vi "Dashboard Main.vi"() -> ()   [LabVIEW 2014]
uses:
  Common Code/Elevator DB Control.ctl
  Common Code/Elevator Presets.ctl
  Common Code/Roller Indicators.ctl
  Common Code/Roller Mode Enum.ctl
  Common Code/Auto Roller Commands.ctl
  Common Code/Inner Roller States.ctl
  Robot Code/Sensors/Pot Data.ctl
  Robot Code/Rollers/Untip Can States.ctl
  Common Code/Roller Control.ctl
  <vilib>/Rock Robotics/WPI/Camera/WPI_CameraSettings Read MJPG.ctl
  <vilib>/Rock Robotics/WPI/Camera/WPI_CameraImageSize.ctl
  Common Code/Encoder Control.ctl
  Common Code/Encoder Values SuperCluster.ctl
  Common Code/Encoder Values.ctl
  Common Code/Power and Diagnostic Data.ctl
  Common Code/Utilities/PDP Data.ctl
  Common Code/Utilities/PCM Data.ctl
  Common Code/Loop Timings.ctl
  Common Code/Ultrasonic Indicators.ctl
  Common Code/Drivetrain Status.ctl
  Robot Code/Drivetrain Code/Drivetrain Mode.ctl
  Common Code/Dist Drive Status.ctl
  Common Code/Yaw Rate Compensation Indicators.ctl
  <vilib>/vision/Image Controls.llb/IMAQ Image.ctl
  Vision/Particle Filter Settings.ctl
  Robot Code/Rollers/ThinRollerIndicators.ctl
  Vision/Vision Tote Data.ctl
  Common Code/commandCluster.ctl
  Common Code/Drivetrain Settings.ctl
  Common Code/IMU Data.ctl
  navX-MXP Library/COMMON/TypeDefs/Value TypeDefs/navX NAVX_CAL_STATUS.ctl
  navX-MXP Library/COMMON/TypeDefs/Value TypeDefs/navX NAVX_OP_STATUS.ctl
  Common Code/Elevator Status.ctl
  Common Code/Elevator Mode.ctl
  Common Code/Auto Elevator Indicators.ctl
  Common Code/Elevator State.ctl
  Robot Code/Pike/Pike Indicators.ctl
  Robot Code/Pike/Pike State.ctl
  Robot Code/Pike/Pike Mode.ctl
  <vilib>/Utility/miscctls.llb/LVPointTypeDef.ctl
  Common Code/Dashboard Control Data.ctl
  Robot Code/Pike/Pike DB Controls.ctl
  Common Code/Dashboard Display Data.ctl
  Common Code/AutonomousDBPacket.ctl
  <vilib>/Rock Robotics/WPI/Dashboard/WPI_DashboardLogging Global.vi
  <vilib>/picture/picture.llb/Draw True-Color Pixmap.vi
  <vilib>/Utility/config.llb/Write Key (String).vi
  <vilib>/Utility/config.llb/Write Key (I32).vi
  <vilib>/Utility/inputDevices.llb/keyboardAcquire.vi
  <vilib>/Utility/config.llb/NI_LVConfig.lvlib
  navX-MXP Library/navX-MXP IMU.lvlib
panel:
  out "Axis Cam":T1
  out "DumbDash Message":string
  in  "Load":bool
  in  "Save":bool
  in  "stop":bool
  in  "TCP":refnum<k5>
  in  "Rec Mode":enum32{"Stop", "Record", "Playback"}(radio)
  out "Camera IP":string
  out "Image Message":string="Timeout in Camera Communications"
  in  "Dashboard Tab":T2(tab)
  out "Pike":bool
  in  "Dallas load":bool
  out "Stabilizer":bool
  out "Finger":bool
  out "NAVX_CAL_STATUS":T3 items=["IMU_CAL_STATE_MASK"=3, "IMU_CAL_INPROGRESS"=0, "IMU_CAL_ACCUMULATE"=1, "IMU_CAL_COMPLETE"=2, "MAG_CAL_COMPLETE"=4, "BARO_CAL_COMPLETE"=8]
  out "Elevator View 2":picture
  out "Trashcan? 2":bool caption="Trashcan?"
  out "Robot Mode":T4(ring)=enum."Auto Disabled"
  out "Gyro":dbl(knob) scale=0.0..360.0 scale format="%#.7g"
  out "Roller Indicators":T5={"Rollers Closed?"=FALSE, "Zero Complete?"=FALSE, "Roller Mode"=enum."Manual", "Auto Roller State"=enum."Grab Tote", "Intake State"=enum."Acquire Tote", "Left Out"=0.0, "Roller Safety Open"=FALSE, "Right Out"=0.0} {"Right Out" scale=-1.0..1.0; "Left Out" scale=-1.0..1.0}
  out "Elevator Mode":bool
  out "Roller Mode":bool
  out "Pressure":dbl format="%#.1f"
  out "Ultrasonic Data 2":T9
  out "Auton File":string
  out "Elevator Status Data 2":T10 {"Finger Raw" format="%#.3f"; "Finger Height" format="%#.3f"; "Motor Out" scale=-1.0..1.0}
  out "Robot IP":string
  out "Pike Indicators":T14={"Motor Out"=0.0, "Current"=0.0, "Limit Switch"=FALSE, "Current Limit"=FALSE, "State"=enum."Going Up", "Command"=enum."Auto Up"}
  out "Auton File Count":i32
  out "Directory":string
  out "Current File":string
  out "File Index":i32
  out "Current Auto Command Data":T17
  out "Drivetrain 4":T18 {"Translation X" scale=-1.0..1.0; "X (Steer)" scale=-1.0..1.0; "Y (Throttle)" scale=-1.0..1.0}
  in  "Mask View":bool
  in  "Camera Settings":T22={"Frame Rate"=30, "Compression"=30, "Size"=1} {"Frame Rate" scale=1.0..30.0; "Size" items=["640x480", "320x240", "160x120"]}
  in  "Camera FOV width":dbl
  in  "Cam Exposure":dbl
  out "Axis Display":T1(plugin-control)
  in  "Vision":u16(ring) items=["Camera Off", "USB Camera SW", "USB Camera HW", "IP Camera"]
  out "Mbps 2":bool
  out "Mbps":dbl format="%#.1g"
  out "fps":dbl format="%#.1g"
  in  "DB Camera Config":bool
  in  "File Path":path
  in  "Use File":bool
  in  "Min target size %":dbl format="%#_13g"
  in  "Camera Settings 2":T23={"fps"=30, "compression"=30, "Image Size"=enum."320x240"}
  out "USB Cam":T1(plugin-control)
  out "fps 2":dbl format="%#.1g"
  out "Mbps 2":dbl format="%#.1g"
  out "Total mbps":dbl
  in  "Filter Settings":T25
  in  "Ring Light Color":T26={"Hue"={101.37467765958063, 64.10933859299683}, "Sat"={88.03571428571429, 255.0}, "Val"={133.57142857142858, 255.0}} {"Hue" scale=0.0..255.0 scale format="%#_3g"}
  out "Detected totes":T27[](array[typedef])
  in  "Camera Mode":u16(ring) items=["Camera Off", "USB Camera SW", "USB Camera HW", "IP Camera"]
  in  "Rectangle":T28
  out "Power and Diagnostic Data":T29
  out "Status Info":T32
  out "Robot Metrics":T33
  out "DS TCP":T34
  out "Control Info":T35
  out "Loop Timings":T36
  out "IMU Gyro":dbl(knob) scale=0.0..360.0 scale format="%#.7g"
  out "Roll":dbl(knob) scale=-90.0..90.0
  out "Pitch":dbl(knob) scale=-90.0..90.0
  in  "Yaw PID Gains":T37={"proportional gain (Kc)"=0.0624, "integral time (Ti, min)"=0.0, "derivative time (Td, min)"=0.002}
  in  "Yaw PID Output Range":cluster{"output high":dbl, "output low":dbl}={"output high"=0.75, "output low"=-0.75}
  in  "Go to angle":dbl
  out "IMU Data":T38 {"NAVX_OP_STATUS" items=["INITIALIZING", "SELFTEST_IN_PROGRESS", "ERROR", "IMU_AUTOCAL_IN_PROGRESS", "NORMAL"]; "NAVX_CAL_STATUS" items=["IMU_CAL_STATE_MASK"=3, "IMU_CAL_INPROGRESS"=0, "IMU_CAL_ACCUMULATE"=1, "IMU_CAL_COMPLETE"=2, "MAG_CAL_COMPLETE"=4, "BARO_CAL_COMPLETE"=8]}
  in  "Drivetrain Settings":T40={"Gyro Tolerance"=0.0, "Strafe Correct max steer"=0.4, "Strafe Timer Wait"=250.0, "Throttle Ramp (ms)"=0.0, "Strafe Ramp (ms)"=0.0, "Angular rate compensation"=FALSE, "Throttle to Rate Scale"=0.0, "Rate compensation gain"=0.0, "Creep Steer"=0.0, "Creep Throttle"=0.0} {"Rate compensation gain" format="%#_6f"; "Throttle to Rate Scale" format="%#_6f"}
  out "Encoder Values":T41 {"Right Encoder"."Ticks" format="%#.6g"; "Center Encoder"."Ticks" format="%#.6g"; "Left Encoder"."Ticks" format="%#.6g"}
  in  "Encoder Control":T43={"Left Tick Constant"=1.0, "Right Tick Constant"=0.0, "Center Tick Constant"=0.0, "Reset?"=FALSE, "Y Dist"={"PID gains"={"proportional gain (Kc)"=1.0, "integral time (Ti, min)"=0.0, "derivative time (Td, min)"=0.0}}, "X Dist"={"PID gains"={"proportional gain (Kc)"=1.0, "integral time (Ti, min)"=0.0, "derivative time (Td, min)"=0.0}}, "Y Stop Thresh"=0.0, "Y Stop Speed"=0.0, "X Stop Thresh"=0.0, "X Stop Speed"=0.0} {"X Dist"."PID gains"."derivative time (Td, min)" format="%.3f"; "X Dist"."PID gains"."integral time (Ti, min)" format="%.3f"; "X Dist"."PID gains"."proportional gain (Kc)" format="%.3f"; "Y Dist"."PID gains"."derivative time (Td, min)" format="%.3f"; "Y Dist"."PID gains"."integral time (Ti, min)" format="%.3f"; "Y Dist"."PID gains"."proportional gain (Kc)" format="%.3f"}
  out "Drivetrain":T18 {"Translation X" scale=-1.0..1.0; "X (Steer)" scale=-1.0..1.0; "Y (Throttle)" scale=-1.0..1.0}
  out "Zeroing Rollers?":bool
  out "Roller State Indicators":T44={"Rollers Closed?"=FALSE, "Roller Mode"=enum."Manual", "Auto Roller State"=enum."Grab Tote", "Tote Inside?"=FALSE, "Intake State"=enum."Acquire Tote", "Left Ping Dist"=0.0, "Right Ping Dist"=0.0, "Potentiometer Cluster"={"Left Pot Zero"=0.0, "Right Pot Zero"=0.0, "Left Potentiometer"=0.0, "Right Potentiometer"=0.0, "Left Pot Non Zero"=0.0, "Right Pot Non Zero"=0.0}, "PING Decision"=enum."Acquire Tote", "Zero Complete?"=FALSE, "Left Arm Closed?"=FALSE, "Portrait?"=FALSE, "Right Arm Closed?"=FALSE, "Left Out"=0.0, "Right Out"=0.0, "Left Current"=0.0, "Right Current"=0.0, "Tote Load Complete?"=FALSE, "Untip Complete?"=FALSE, "Untip State"=enum."Idle", "Roller Safety Open"=FALSE} {"Right Out" scale=-1.0..1.0; "Left Out" scale=-1.0..1.0}
  in  "Roller Settings":T47={"Intake Speed"=0.7, "Turn In Speed"=0.7, "Unload Speed"=-0.7, "Turn Out Speed"=-0.7, "Ping Align Tolerance"=1000.0, "Tote Range Threshold"=0.0, "Right Pot 0"=0.0, "Pot Threshold"=0.0, "Left Pot 0"=0.0, "Manual 0s?"=FALSE, "Right Pot Scale"=0.0, "Left Pot Scale"=0.0, "0 wait time"=0, "Zero Pots"=FALSE, "Min Elevator Height"=0.0, "Eject Time"=0.0, "Eject US Threshold"=0.0, "Anti-Twitch Time"=0, "Ping Caring Threshold"=0.0, "Pot Diff Threshold"=0.0, "Pinch Sustain"=0, "Absorb Give Up Threshold"=0.0, "Untip In Threshold"=0.0, "Untip Grab Range"=0.0, "Ultrasonic Hold Time"=0, "Landscape Absorb Time"=0, "Pot Use Wait Time"=0, "Can Turn Stop Range"=0.0, "Ignore Pressure"=FALSE, "HP Load Speed"=0.0}
  out "Ultrasonic Data":T9
  in  "Pressure m Value":dbl=34.774
  in  "Pressure b Value":dbl=-58.564
  out "Transducer Voltage":dbl
  out "Pressure 2":dbl
  out "Trashcan?":bool
  out "Tote Count":i32
  in  "Elevator":T48={"PID Output Range"={"output high"=1.0, "output low"=-1.0}, "PID gains"={"proportional gain (Kc)"=1.0, "integral time (Ti, min)"=0.0, "derivative time (Td, min)"=0.0}, "Height Tolerance"=0.5, " Encoder Constant"=0.0027952480782669, "Safe Mode Max Speed"=0.0, "Eject Time"=0.0, "Zeroing Speed"=1.0, "Presets"={"Pickup 2 w/ Tote"=27.0, "Pickup 2 w/ Trashcan"=25.0, "Pickup 3 w/ Tote"=40.0, "Pickup 3 w/ Trashcan"=25.0, "Bottom"=0.0, "Pickup 1 w/ Tote"=17.0, "Pickup Trashcan"=0.0, "Pickup 1 w/ Trashcan"=25.0, "Eject"=0.0, "Hold Low"=0.0, "Step add height"=0.0, "Untip Lift"=0.0, "Drop Stack"=0.0, "HP Load Hold"=0.0, "HP Load Drop"=0.0, "HP Load Finger"=0.0, "HP Load Hold Can"=0.0, "Store can max"=0.0, "HP Drag Score"=0.0, "HP Store can max"=0.0, "HP Drag Finish"=0.0, "HP Carry min"=0.0, "HP Finger Anti-Crash"=0.0, "Finger trashcan avoid"=0.0}, "Ping Detect Threshold"=0.0, "Trashcan Detect Threshold"=0.0, "Zero Filter Time"=0.0, "Stabilizer Open Time"=0.0, "Zero Creep Speed"=0.0, "Max Current"=0.0, "Current Trip Time"=0.0, "Abort Pitch"=0.0, "Finger m"=0.0, "Finger b"=0.0, "Finger max "=0.0, "Finger Stabilizer"=0.0, "Finger Store"=0.0, "Finger Stop Store"=0.0, "Stabilizer Close Time"=0.0, "HP Finger Store"=0.0, "HP Finger Stop Store"=0.0, "Finger min"=0.0, "Unstick gain"=0.0, "Roller Wait"=0.0} {"Encoder Constant" format="%.6f"}
  out "Ultrasonic Data 3":T9
  out "Elevator Status Data 3":T10 {"Motor Out" scale=-1.0..1.0}
  # "Steering PID"
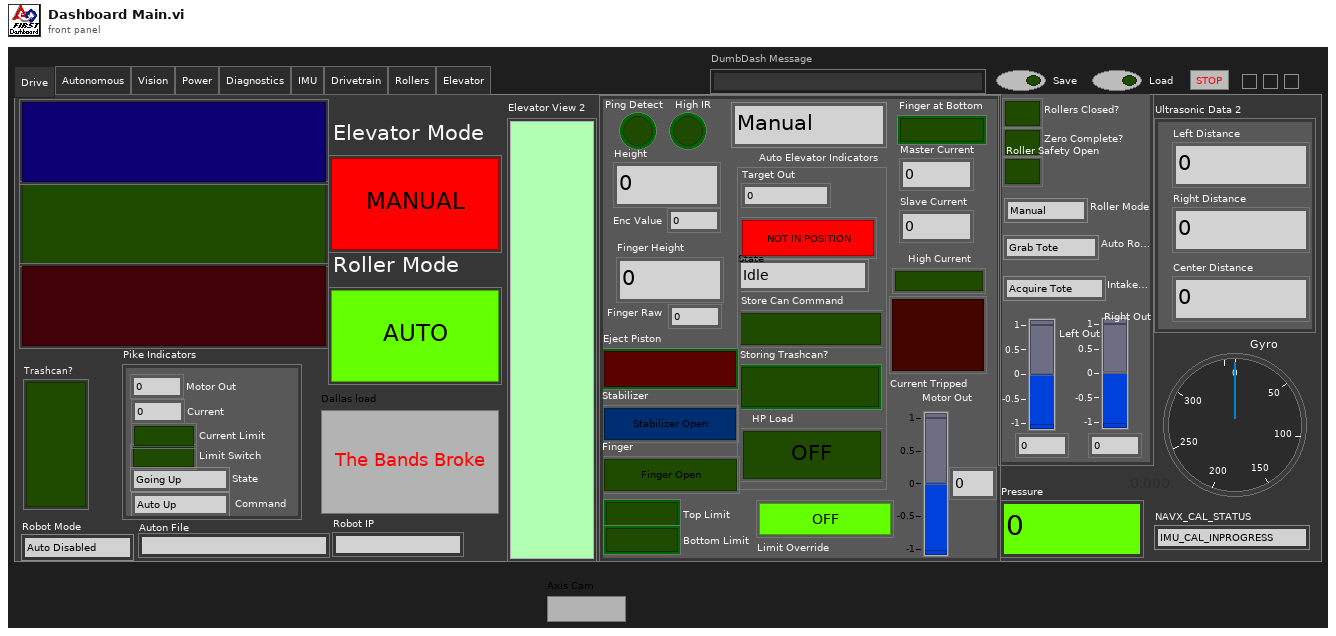
[diagram p1: front panel]
types:
  T1 = typedef "IMAQ Image.ctl" = refnum<image>
  T2 = enum32{"Drive", "Autonomous", "Vision", "Power", "Diagnostics", "IMU", "Drivetrain", "Rollers", "Elevator"}
  T3 = typedef "navX-MXP IMU.lvlib/navX NAVX_CAL_STATUS.ctl" = u8
  T4 = enum8{"Tele-Op Disabled", "Tele-Op Enabled", "Auto Disabled", "Auto Enabled", "Test Disabled", "Test Enabled", "Disconnected", "No Code", "E-Stop"}
  T5 = typedef "ThinRollerIndicators.ctl" = cluster{"Rollers Closed?":bool, "Zero Complete?":bool, "Roller Mode":T6, "Auto Roller State":T7, "Intake State":T8, "Left Out":dbl, "Roller Safety Open":bool, "Right Out":dbl}
  T6 = typedef "Roller Mode Enum.ctl" = enum16{"Manual", "Safe", "Auto"}
  T7 = typedef "Auto Roller Commands.ctl" = enum16{"Drag Tote", "Grab Tote", "Idle", "Eject Tote", "Untip Can", "Grab Can"}
  T8 = typedef "Inner Roller States.ctl" = enum16{"Turn Tote Portrait", "Acquire Tote", "Absorb Tote", "Turn Tote Right", "Turn Tote Left", "Acquire Can", "Absorb Can", "Turn Can", "Hold Tote"}
  T9 = typedef "Ultrasonic Indicators.ctl" = cluster{"Left Distance":dbl, "Right Distance":dbl, "Center Distance":dbl, "Left Distance Unfilter":dbl, "Right Distance Unfilter":dbl, "Center Distance Unfilter":dbl}
  T10 = typedef "Elevator Status.ctl" = cluster{"Height":dbl, "Enc Value":dbl, "Limit Override":bool, "Mode":T11, "High IR":bool, "Motor Out":dbl, "Ping Detect":bool, "Auto Elevator Indicators":T12, "Master Current":dbl, "Slave Current":dbl, "High Current":bool, "Current Tripped":bool, "Top Limit":bool, "Bottom Limit":bool, "Eject Piston":bool, "Stabilizer":bool, "Finger":bool, "Finger Height":dbl, "Finger Raw":dbl, "Finger at Bottom":bool}
  T11 = typedef "Elevator Mode.ctl" = enum16{"Manual", "Safe", "Auto"}
  T12 = typedef "Auto Elevator Indicators.ctl" = cluster{"Target Out":dbl, "Storing Trashcan?":bool, "State":T13, "In Range":bool, "Store Can Command":bool, "HP Load":bool}
  T13 = typedef "Elevator State.ctl" = enum16{"Idle", "Goto Load Position", "Wait for Load", "Load Drop", "Load Lift", "Drop Stack", "Goto Eject Position", "Eject ", "Raise Trashcan", "Open Stabilizer", "Untip Drop", "Untip Wait", "Untip Lift", "Abort Load", "HP Load Wait", "HP Load Drop", "HP Load Lift", "HP Load Abort", "Close Stabilizer", "HP Load Lift First Tote", "HP Load Drop First Tote", "HP Load Unfinish", "HP Drag Score", "HP Drag Finish Up", "HP Drag Finish Down", "HP Carry Finish Drop", "HP Carry Finish Lift", "HP Carry Score"}
  T14 = typedef "Pike Indicators.ctl" = cluster{"Motor Out":dbl, "Current":dbl, "Limit Switch":bool, "Current Limit":bool, "State":T15, "Command":T16}
  T15 = typedef "Pike State.ctl" = enum16{"Up", "Down", "Going Up", "Going Down"}
  T16 = typedef "Pike Mode.ctl" = enum16{"Idle", "Auto Down", "Auto Up", "Manual Down", "Manual Up"}
  T17 = typedef "commandCluster.ctl" = cluster{"Step ID":i16, "Command Type":i16, "Drive X":sgl, "Drive Y":sgl, "Heading":sgl, "Max Exec. Time":i16, "Jump Type":i32, "Jump To":i16, "Jump Condition":i16, "Async Drive?":i16, "Roller Mode":i16, "Roller Align":i16, "Roller Closed?":i16, "Wait Condition":i16, "Elevator Mode":i16, "Elevator Command":i16, "Roller State":i16, "Hold Low?":i16, "Num Totes":i16, "Num Cans":dbl, "Past Distance":dbl, "Store Can?":dbl, "X Speed":dbl, "Y Speed":dbl, "Yaw Angle Set":dbl, "Grab Can":dbl, "Roller Overide Speed":dbl, "Force Load?":sgl, "Set Idle":sgl, "Eject":sgl, "Pike Action":sgl}
  T18 = typedef "Drivetrain Status.ctl" = cluster{"Y (Throttle)":sgl, "X (Steer)":sgl, "Translation X":sgl, "Center Wheel Down":bool, "Mode":T19, "Distance Drive finished?":bool, "Y Target":sgl, "X Target":sgl, "Heading Target":sgl, "Dist Drive Status":T20, "Step Eject Lockout":bool, "Gyro In Range?":bool, "Yaw Comp Indicators":T21}
  T19 = typedef "Drivetrain Mode.ctl" = enum16{"Manual", "Gyro Steer", "Vision Steer", "Drive Distance", "Yaw Rate Compensate"}
  T20 = typedef "Dist Drive Status.ctl" = cluster{"Y In Range":bool, "X In Range":bool, "Gyro In Range":bool, "Y Dist":dbl, "X Dist":dbl, "Gyro":dbl}
  T21 = typedef "Yaw Rate Compensation Indicators.ctl" = cluster{"Rate Command":sgl, "Rate Actual":sgl, "Steer adjustment":sgl}
  T22 = cluster{"Frame Rate":i32, "Compression":i32, "Size":u16}
  T23 = typedef "WPI_CameraSettings Read MJPG.ctl" = cluster{"fps":i32, "compression":i32, "Image Size":T24}
  T24 = typedef "WPI_CameraImageSize.ctl" = enum16{"640x480", "320x240", "160x120", "Custom"}
  T25 = typedef "Particle Filter Settings.ctl" = cluster{"Min Aspect Score":dbl, "Min Area Score":dbl, "Min X Score":dbl, "Min Y Score":dbl}
  T26 = cluster{"Hue":cluster{dbl, dbl}, "Sat":cluster{dbl, dbl}, "Val":cluster{dbl, dbl}}
  T27 = typedef "Vision Tote Data.ctl" = cluster{"Left _|":cluster{"Bounding box":cluster{"left":dbl, "top":dbl, "right":dbl, "bottom":dbl}, "Aspect Ratio":dbl, "Area Score":dbl, "X Mask":dbl, "Y Mask":dbl, "Ell":bool}, "Right |_":cluster{"Bounding box":cluster{"left":dbl, "top":dbl, "right":dbl, "bottom":dbl}, "Aspect Ratio":dbl, "Area Score":dbl, "X Mask":dbl, "Y Mask":dbl, "Ell":bool}, "Center X":dbl, "Center Y":dbl, "Angle Offset":dbl}
  T28 = cluster{"Left":i32, "Top":i32, "Right":i32, "Bottom":i32}
  T29 = typedef "Power and Diagnostic Data.ctl" = cluster{"PDP Data":T30, "PCM Data":T31, "roboRIO input voltage (V)":dbl, "roboRIO input current (A)":dbl, "3.3V Rail Short":bool, "5 V Rail Short":bool, "6 V Rail Short":bool, "roboRIO Brownout":bool, "Outputs Enabled?":bool}
  T30 = typedef "PDP Data.ctl" = cluster{"Battery Voltage":sgl, "Temperature (degrees C)":sgl, "Internal Battery R (Ohms)":sgl, "Energy (J)":sgl, "Power (W)":sgl, "Total Current (A)":sgl, "Battery Voltage Fault":bool, "Temperature Fault":bool, "Hardware Fault":bool, "Currents":cluster{"[0]":sgl, "[1]":sgl, "[2]":sgl, "[3]":sgl, "[4]":sgl, "[5]":sgl, "[6]":sgl, "[7]":sgl, "[8]":sgl, "[9]":sgl, "[10]":sgl, "[11]":sgl, "[12]":sgl, "[13]":sgl, "[14]":sgl, "[15]":sgl}, "Current Faults":cluster{"[0]":bool, "[1]":bool, "[2]":bool, "[3]":bool, "[4]":bool, "[5]":bool, "[6]":bool, "[7]":bool, "[8]":bool, "[9]":bool, "[10]":bool, "[11]":bool, "[12]":bool, "[13]":bool, "[14]":bool, "[15]":bool}}
  T31 = typedef "PCM Data.ctl" = cluster{"Compressor Fault":bool, "Solenoid Fault":bool, "Compressor Enabled":bool, "Hardware Fault":bool, "Compressor Current":dbl}
  T32 = cluster{"Status bits":cluster{"Test Mode":bool, "Autonomous":bool, "Enabled":bool, "Code Start":bool, "Brownout":bool, "Reserved 2":bool, "Reserved 3":bool, "E-Stop":bool}, "Code Trace":cluster{"Disabled":bool, "TeleOp":bool, "Auto":bool, "Test":bool}, "Controller Type":enum16{"unknown", "cRIO", "roboRio"}, "Code?":enum16{"unknown", "noCode", "code"}, "Battery V":dbl}
  T33 = cluster{"Storage":cluster{"Disk Free":u64, "RAM Block":u32, "RAM free":u32}, "CPU Utilization":cluster{"CPU % ISR":sgl, "CPU % Time Crit":sgl, "CPU % Timed Str":sgl, "CPU % High":sgl, "CPU % Above":sgl, "CPU % Normal":sgl, "CPU % Low":sgl}, "CAN":cluster{"% Bus Utilization":sgl, "Bus Off Cnt":u32, "TX_FIFO Full Cnt":u32, "Receive Error Cnt":u8, "Transmit Error Cnt":u8}, "HID":cluster{"HID Outputs":u32, "Rumble Low":u16, "Rumble High":u16}[]}
  T34 = cluster{"Error Strings":string, "Disable Counts":cluster{u16, u16}, "Rail Faults":cluster{u16, u16, u16}, "Robot IP":string, "DB Mode":u8, "Event Info":cluster{"Name":string, "Type":u8, "Number":u16, "Replay":u8}, "Camera Addr":string}
  T35 = cluster{"Control Bits":cluster{"TestMode":bool, "Autonomous":bool, "Enabled":bool, "FMS Present":bool, bool, bool, bool, "E-Stop":bool}, "Team Station ":u8, "Countdown":sgl, "Joystick Values":cluster{"Axes":dbl[], "Buttons":bool[], "POVs":i16[]}[]}
  T36 = typedef "Loop Timings.ctl" = cluster{"Roller Loop":i32, "Elevator Loop":i32, "US Loop":i32, "100ms Loop":i32, "Drivetrain Loop":i32}
  T37 = cluster{"proportional gain (Kc)":dbl, "integral time (Ti, min)":dbl, "derivative time (Td, min)":dbl}
  T38 = typedef "IMU Data.ctl" = cluster{"Pitch":sgl, "Roll":sgl, "Yaw":sgl, "Data Valid?":bool, "Temp":sgl, "MOVING":bool, "NAVX_CAL_STATUS":T3, "NAVX_OP_STATUS":T39, "YAW_STABLE":bool, "Accel X":sgl, "Accel Y":sgl, "Accel Z":sgl, "Accel Magnitude":sgl, "Pitch Rate":sgl, "Roll Rate":sgl, "Yaw Rate":sgl, "NavX Opened?":bool}
  T39 = typedef "navX-MXP IMU.lvlib/navX NAVX_OP_STATUS.ctl" = u8
  T40 = typedef "Drivetrain Settings.ctl" = cluster{"Gyro Tolerance":sgl, "Strafe Correct max steer":sgl, "Strafe Timer Wait":sgl, "Throttle Ramp (ms)":sgl, "Strafe Ramp (ms)":sgl, "Angular rate compensation":bool, "Throttle to Rate Scale":sgl, "Rate compensation gain":sgl, "Creep Steer":sgl, "Creep Throttle":sgl}
  T41 = typedef "Encoder Values SuperCluster.ctl" = cluster{"Left Encoder":T42, "Center Encoder":T42, "Right Encoder":T42}
  T42 = typedef "Encoder Values.ctl" = cluster{"Distance":dbl, "Speed":dbl, "Ticks":dbl}
  T43 = typedef "Encoder Control.ctl" = cluster{"Left Tick Constant":dbl, "Right Tick Constant":dbl, "Center Tick Constant":dbl, "Reset?":bool, "Y Dist":cluster{"PID gains":cluster{"proportional gain (Kc)":dbl, "integral time (Ti, min)":dbl, "derivative time (Td, min)":dbl}}, "X Dist":cluster{"PID gains":cluster{"proportional gain (Kc)":dbl, "integral time (Ti, min)":dbl, "derivative time (Td, min)":dbl}}, "Y Stop Thresh":dbl, "Y Stop Speed":dbl, "X Stop Thresh":dbl, "X Stop Speed":dbl}
  T44 = typedef "Roller Indicators.ctl" = cluster{"Rollers Closed?":bool, "Roller Mode":T6, "Auto Roller State":T7, "Tote Inside?":bool, "Intake State":T8, "Left Ping Dist":sgl, "Right Ping Dist":sgl, "Potentiometer Cluster":T45, "PING Decision":T8, "Zero Complete?":bool, "Left Arm Closed?":bool, "Portrait?":bool, "Right Arm Closed?":bool, "Left Out":sgl, "Right Out":sgl, "Left Current":sgl, "Right Current":sgl, "Tote Load Complete?":bool, "Untip Complete?":bool, "Untip State":T46, "Roller Safety Open":bool}
  T45 = typedef "Pot Data.ctl" = cluster{"Left Pot Zero":sgl, "Right Pot Zero":sgl, "Left Potentiometer":sgl, "Right Potentiometer":sgl, "Left Pot Non Zero":sgl, "Right Pot Non Zero":sgl}
  T46 = typedef "Untip Can States.ctl" = enum16{"Release Can", "Catch Can", "Idle"}
  T47 = typedef "Roller Control.ctl" = cluster{"Intake Speed":dbl, "Turn In Speed":dbl, "Unload Speed":dbl, "Turn Out Speed":dbl, "Ping Align Tolerance":dbl, "Tote Range Threshold":dbl, "Right Pot 0":dbl, "Pot Threshold":dbl, "Left Pot 0":dbl, "Manual 0s?":bool, "Right Pot Scale":dbl, "Left Pot Scale":dbl, "0 wait time":i32, "Zero Pots":bool, "Min Elevator Height":dbl, "Eject Time":dbl, "Eject US Threshold":dbl, "Anti-Twitch Time":u32, "Ping Caring Threshold":dbl, "Pot Diff Threshold":dbl, "Pinch Sustain":u32, "Absorb Give Up Threshold":dbl, "Untip In Threshold":dbl, "Untip Grab Range":dbl, "Ultrasonic Hold Time":u32, "Landscape Absorb Time":u32, "Pot Use Wait Time":u32, "Can Turn Stop Range":dbl, "Ignore Pressure":bool, "HP Load Speed":dbl}
  T48 = typedef "Elevator DB Control.ctl" = cluster{"PID Output Range":cluster{"output high":dbl, "output low":dbl}, "PID gains":cluster{"proportional gain (Kc)":dbl, "integral time (Ti, min)":dbl, "derivative time (Td, min)":dbl}, "Height Tolerance":sgl, " Encoder Constant":dbl, "Safe Mode Max Speed":sgl, "Eject Time":sgl, "Zeroing Speed":sgl, "Presets":T49, "Ping Detect Threshold":sgl, "Trashcan Detect Threshold":sgl, "Zero Filter Time":dbl, "Stabilizer Open Time":dbl, "Zero Creep Speed":dbl, "Max Current":dbl, "Current Trip Time":dbl, "Abort Pitch":dbl, "Finger m":dbl, "Finger b":dbl, "Finger max ":dbl, "Finger Stabilizer":dbl, "Finger Store":dbl, "Finger Stop Store":dbl, "Stabilizer Close Time":dbl, "HP Finger Store":dbl, "HP Finger Stop Store":dbl, "Finger min":dbl, "Unstick gain":dbl, "Roller Wait":dbl}
  T49 = typedef "Elevator Presets.ctl" = cluster{"Pickup 2 w/ Tote":sgl, "Pickup 2 w/ Trashcan":sgl, "Pickup 3 w/ Tote":sgl, "Pickup 3 w/ Trashcan":sgl, "Bottom":sgl, "Pickup 1 w/ Tote":sgl, "Pickup Trashcan":sgl, "Pickup 1 w/ Trashcan":sgl, "Eject":sgl, "Hold Low":sgl, "Step add height":sgl, "Untip Lift":dbl, "Drop Stack":dbl, "HP Load Hold":dbl, "HP Load Drop":dbl, "HP Load Finger":dbl, "HP Load Hold Can":dbl, "Store can max":dbl, "HP Drag Score":dbl, "HP Store can max":dbl, "HP Drag Finish":dbl, "HP Carry min":dbl, "HP Finger Anti-Crash":dbl, "Finger trashcan avoid":dbl}
  T50 = typedef "Image Type" = u32
  T51 = enum32{"Invalid", "Standard", "Closed", "Hidden", "Minimized", "Maximized"}
  T52 = typedef "LVPointTypeDef.ctl" = cluster{"Horizontal":i16, "Vertical":i16}
  T53 = typedef "Dashboard Display Data.ctl" = cluster{"Gyro Angle":dbl, "Autonomous":T54, "Pressure Transducer V":dbl, "Pressure":dbl, "Roller State Indicators":T44, "Elevator Status Data":T10, "IMU Data":T38, "Tote Count":i8, "Have Trashcan":bool, "Encoder Values":T41, "Power and Diagnostic Data":T29, "Loop Timings":T36, "Ultrasonic Data":T9, "Zeroing Rollers?":bool, "Drivetrain":T18, "Current Auto Command Data":T17, "Can Grabber":bool, "Pike":T14}
  T54 = typedef "AutonomousDBPacket.ctl" = cluster{"Selected File":string, "Directory":string, "Auton File Index":i32, "Auton File Count":i32, "Auton Command Array":T17[]}
  T55 = typedef "NI_LVConfig.lvlib/Config Data RefNum.ctl" = refnum<k1>
  T56 = cluster{"Image Size":bool, "Image Type":bool, "Pixel Value":bool, "ROI Information":bool, "Zoom Factor":bool}
  T57 = enum8{"Enabled", "Disabled", "Disabled and Grayed Out"}
  T58 = enum16{"0", "1", "2", "3", "4", "5", "6", "7", "8", "9", "A", "B", "C", "D", "E", "F", "G", "H", "I", "J", "K", "L", "M", "N", "O", "P", "Q", "R", "S", "T", "U", "V", "W", "X", "Y", "Z", "F1", "F2", "F3", "F4", "F5", "F6", "F7", "F8", "F9", "F10", "F11", "F12", "F13", "F14", "F15", "ADD", "BACK", "BACKSLASH", "CAPITAL", "COMMA", "DECIMAL", "DELETE", "DIVIDE", "DOWN", "END", "EQUALS", "ESCAPE", "GRAVE (`)", "HOME", "INSERT", "LBRACKET", "LCONTROL", "LEFT", "L ALT", "LSHIFT", "LWIN", "MINUS", "MULTIPLY", "NEXT", "NUMLOCK", "NUMPAD_0", "NUMPAD_1", "NUMPAD_2", "NUMPAD_3", "NUMPAD_4", "NUMPAD_5", "NUMPAD_6", "NUMPAD_7", "NUMPAD_8", "NUMPAD_9", "PAUSE", "PERIOD", "PRIOR (PG UP)", "RBRACKET", "RCONTROL", "RETURN", "RIGHT", "R ALT", "RSHIFT", "RWIN", "SCROLL", "SEMICOLON", "SLASH", "SPACE", "SUBTRACT", "TAB", "UP", "ENTER (num pad)", "' (quote)"}[]
  T59 = typedef "Dashboard Control Data.ctl" = cluster{"Cam Exposure":dbl, "Go to angle":dbl, "Steer PID Gains":cluster{"proportional gain (Kc)":dbl, "integral time (Ti, min)":dbl, "derivative time (Td, min)":dbl}, "Steer PID output Range":cluster{"output high":dbl, "output low":dbl}, "Pressure m \nValue":dbl, "Pressure b \nValue":dbl, "Roller Command Cluster ":T47, "Elevator":T48, "Encoder Control":T43, "Auton Settings":cluster{"Drive Dist Window Size":dbl}, "Drivetrain Settings":T40, "Lance":T60}
  T60 = typedef "Pike DB Controls.ctl" = cluster{"Down Speed":dbl, "Up Speed":dbl, "Max Down Time":dbl, "Max Up Time":dbl, "Current Limit":dbl}
  T61 = typedef "DumbDash Control.ctl" = cluster{"Name":string, "Ref":refnum<vi>, "Type":T62}
  T62 = typedef "DumbDash Control Type.ctl" = enum16{"Invalid", "Number", "Boolean", "String"}
  T63 = typedef "imagedata.ctl" = cluster{"image type":i32, "image depth":i32, "image":u8[], "mask":u8[], "colors":u32[], "Rectangle":cluster{"left":i16, "top":i16, "right":i16, "bottom":i16}}
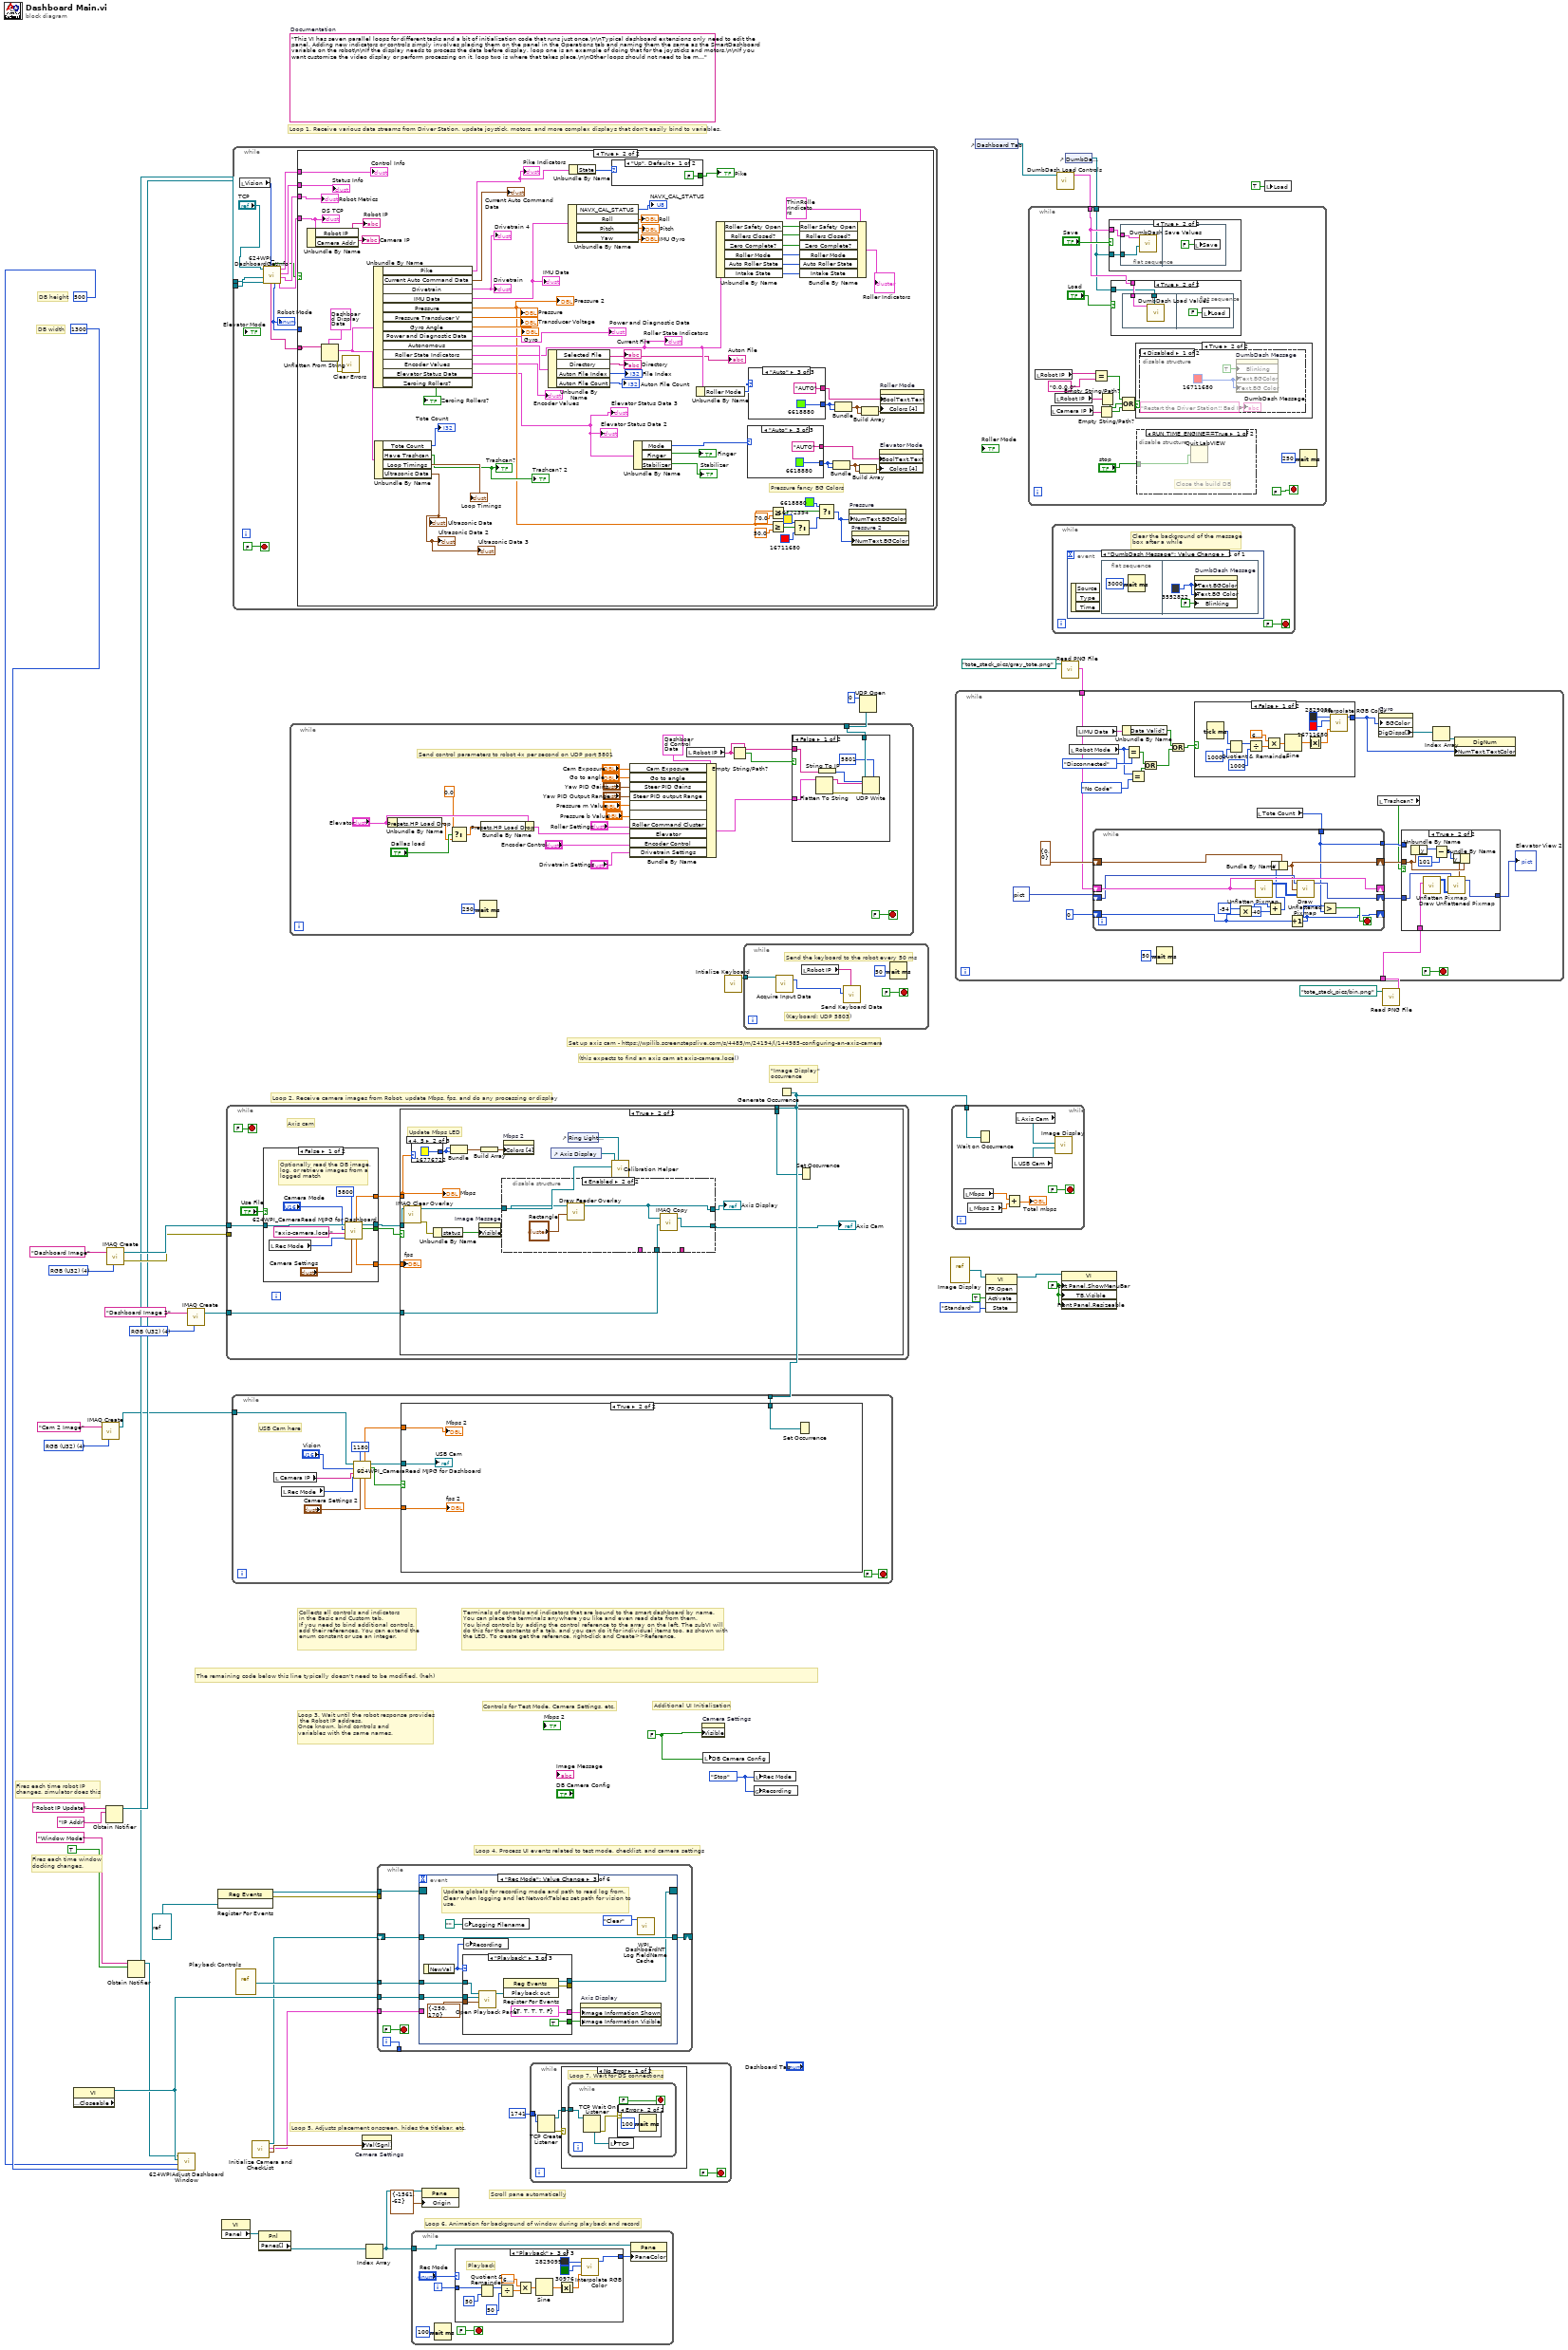
[diagram p0: block diagram]
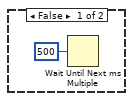
[diagram p4: hidden frame]
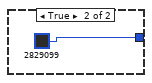
[diagram p5: hidden frame]
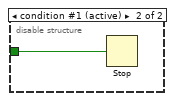
[diagram p8: hidden frame]
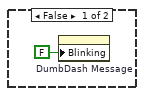
[diagram p9: hidden frame]
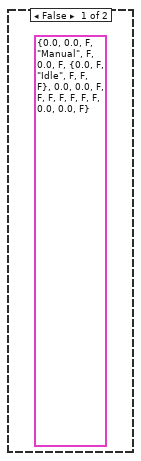
[diagram p13: hidden frame]
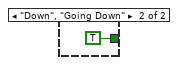
[diagram p14: hidden frame]
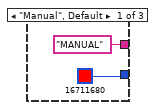
[diagram p15: hidden frame]
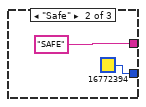
[diagram p16: hidden frame]
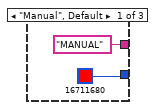
[diagram p17: hidden frame]
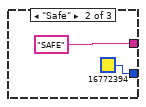
[diagram p18: hidden frame]
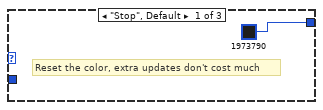
[diagram p19: hidden frame]
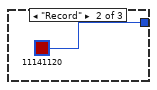
[diagram p20: hidden frame]
diagram:
  w3 = T50 4 items=["Grayscale (U8)", "Grayscale (I16)", "Grayscale (SGL)", "Complex (CSG)", "RGB (U32)", "HSL (U32)", "RGB (U64)"] ("Image Type")
  w6 = FALSE ("Front Panel Window:Show Menu Bar")
  w16 = T50 4 items=["Grayscale (U8)", "Grayscale (I16)", "Grayscale (SGL)", "Complex (CSG)", "RGB (U32)", "HSL (U32)", "RGB (U64)"] ("Image Type")
  w36 = enum32{"Stop", "Record", "Playback"}."Stop" ("Rec Mode")
  w34 = FALSE ("Visible")
  (unwired) "This VI has seven parallel loops for different tasks and a bit of initialization code that runs just once.\n\nTypical dashboard extensions only need to edit the panel. Adding new indicators or controls simply involves placing them on the panel in the Operations tab and naming them the same as the SmartDashboard variable on the robot\n\nIf the display needs to process the data before display, loop one is an example of doing that for the joysticks and motors.\n\nIf you want customize the video display or perform processing on it, loop two is where that takes place.\n\nOther loops should not need to be modified. They are pretty standard, and document the task they perform."  # Documentation
  w50 = T50 4 items=["Grayscale (U8)", "Grayscale (I16)", "Grayscale (SGL)", "Complex (CSG)", "RGB (U32)", "HSL (U32)", "RGB (U64)"] ("Image Type")
  # "\"Image Display\"\noccurrence"
  # "(this expects to find an axis cam at axis-camera.local)"
  # "Set up axis cam - https://wpilib.screenstepslive.com/s/4485/m/24194/l/144985-configuring-an-axis-camera"
  # "Scroll pane automatically"
  # "DB height"
  # "DB width"
  # "Controls for Test Mode, Camera Settings, etc."
  # "Additional UI Initialization"
  # "Loop 6. Animation for background of window during playback and record"
  # "Fires each time robot IP\nchanges, simulator does this"
  # "Fires each time window\ndocking changes."
  # "Collects all controls and indicators\nin the Basic and Custom tab.\nIf you need to bind additional controls,\nadd their references. You can extend the\nenum constant or use an integer."
  # "The remaining code below this line typically doesn't need to be modified. (heh)"
  # "Loop 4. Process UI events related to test mode, checklist, and camera settings"
  # "Terminals of controls and indicators that are bound to the smart dashboard by name.\nYou can place the terminals anywhere you like and even read data from them.\nYou bind controls by adding the control reference to the array on the left. The subVI will\ndo this for the contents of a tab, and you can do it for individual items too, as shown with\nthe LED. To create get the reference, right-click and Create>>Reference."
  # "Loop 3. Wait until the robot response provides\n the Robot IP address.\nOnce known, bind controls and\nvariables with the same names."
  # "Loop 5. Adjusts placement onscreen, hides the titlebar, etc."
  # "Loop 1. Receive various data streams from Driver Station, update joystick, motors, and more complex displays that don't easily bind to variables."
  # "Loop 2. Receive camera images from Robot, update Mbps, fps, and do any processing or display"
  n1 = property class="VI" props=["Front Panel.Closeable"]() -> (reference out=w35:refnum<vi>)  [unwired: 2 in, 2 out]
  n2 = call "IMAQ Create"("Image Name"="Cam 2 Image", "Image Type"=w16) -> ("New Image"=w15:T1)  [unwired: 2 in, 2 out]
  n3 = Obtain Notifier(name (unnamed)="Robot IP Update", notification data type="IP Addr" ("name (unnamed)")) -> (notifier out=w33:refnum<notifier>)  [unwired: 2 in, 2 out]
  n4 = call "IMAQ Create"("Image Name"="Dashboard Image", "Image Type"=w50) -> ("New Image"=w48:T1, "error out"=w47:errorcluster)  [unwired: 2 in, 1 out]
  n5 = Obtain Notifier(name (unnamed)="Window Mode", notification data type=TRUE) -> (notifier out=w32:refnum<notifier>)  [unwired: 2 in, 2 out]
  n6 = call "624WPIAdjust Dashboard Window.vi"("Width"=i16 1300, "Height"=i16 500, "VI"=w35, "Notifier in"=w32) -> ()  [unwired: 8 in]
  n7 = call "IMAQ Create"("Image Name"="Dashboard Image 2", "Image Type"=w3) -> ("New Image"=w1:T1)  [unwired: 2 in, 2 out]
  n8 = register-events(refnum<vi> refnum) -> (reference out=w39:refnum<event-registration>, error out=w38:errorcluster)  [unwired: 2 in]
  n9 = property class="VI"() -> ("Panel"=w41:refnum<vi>)  [unwired: 2 in, 2 out]
  n10 = while {
    tunnel: w33 -> [w61]
    tunnel: w32 -> [w60]
    stop <- FALSE stop-if-true
    n11 = local read "Vision"() -> (w59:u16)
    n12 = call "624WPI_DashboardGetInfo.vi"("Vision"=w59, "Binding Refnum"=w61, "Window Mode Notifier"=w60, "TCP Cnx"="TCP") -> ("Power and Errors"=w57:T34, "Robot Metrics"=w56:T33, "Status Info"=w55:T32, "Control Info"=w54:T35, "Robot Mode"=w53:T4, "Process?"=w51:bool, "Custom Dashboard Data"=w52:string)  [unwired: 1 in]
    "Robot Mode" <- w53
    n13 = case shown="True" w51 {
      tunnel: w55 -> [_ w128]
      tunnel: w56 -> [_ w123]
      tunnel: w54 -> [_ w122]
      tunnel: w57 -> [_ w127]
      tunnel: w53 -> [_ _]
      tunnel: w52 -> [_ w125]
      frame False {
        (unwired) T10 {"Height"=0.0, "Enc Value"=0.0, "Limit Override"=FALSE, "Mode"=enum."Manual", "High IR"=FALSE, "Motor Out"=0.0, "Ping Detect"=FALSE, "Auto Elevator Indicators"={"Target Out"=0.0, "Storing Trashcan?"=FALSE, "State"=enum."Idle", "In Range"=FALSE, "Store Can Command"=FALSE, "HP Load"=FALSE}, "Master Current"=0.0, "Slave Current"=0.0, "High Current"=FALSE, "Current Tripped"=FALSE, "Top Limit"=FALSE, "Bottom Limit"=FALSE, "Eject Piston"=FALSE, "Stabilizer"=FALSE, "Finger"=FALSE, "Finger Height"=0.0, "Finger Raw"=0.0, "Finger at Bottom"=FALSE} ("Elevator Status Data")
      }
      frame True {
        # "Pressure fancy BG Colors"
        n14 = Unbundle By Name(w127) -> ("Robot IP"=→"Robot IP":string, "Camera Addr"=→"Camera IP":string)
        n15 = Unflatten From String(type=T53 {"Gyro Angle"=0.0, "Autonomous"={"Selected File"="", "Directory"="", "Auton File Index"=0, "Auton File Count"=0, "Auton Command Array"=[]}, "Pressure Transducer V"=0.0, "Pressure"=0.0, "Roller State Indicators"={"Rollers Closed?"=FALSE, "Roller Mode"=enum."Manual", "Auto Roller State"=enum."Grab Tote", "Tote Inside?"=FALSE, "Intake State"=enum."Acquire Tote", "Left Ping Dist"=0.0, "Right Ping Dist"=0.0, "Potentiometer Cluster"={"Left Pot Zero"=0.0, "Right Pot Zero"=0.0, "Left Potentiometer"=0.0, "Right Potentiometer"=0.0, "Left Pot Non Zero"=0.0, "Right Pot Non Zero"=0.0}, "PING Decision"=enum."Acquire Tote", "Zero Complete?"=FALSE, "Left Arm Closed?"=FALSE, "Portrait?"=FALSE, "Right Arm Closed?"=FALSE, "Left Out"=0.0, "Right Out"=0.0, "Left Current"=0.0, "Right Current"=0.0, "Tote Load Complete?"=FALSE, "Untip Complete?"=FALSE, "Untip State"=enum."Idle", "Roller Safety Open"=FALSE}, "Elevator Status Data"={"Height"=0.0, "Enc Value"=0.0, "Limit Override"=FALSE, "Mode"=enum."Manual", "High IR"=FALSE, "Motor Out"=0.0, "Ping Detect"=FALSE, "Auto Elevator Indicators"={"Target Out"=0.0, "Storing Trashcan?"=FALSE, "State"=enum."Idle", "In Range"=FALSE, "Store Can Command"=FALSE, "HP Load"=FALSE}, "Master Current"=0.0, "Slave Current"=0.0, "High Current"=FALSE, "Current Tripped"=FALSE, "Top Limit"=FALSE, "Bottom Limit"=FALSE, "Eject Piston"=FALSE, "Stabilizer"=FALSE, "Finger"=FALSE, "Finger Height"=0.0, "Finger Raw"=0.0, "Finger at Bottom"=FALSE}, "IMU Data"={"Pitch"=0.0, "Roll"=0.0, "Yaw"=0.0, "Data Valid?"=FALSE, "Temp"=0.0, "MOVING"=FALSE, "NAVX_CAL_STATUS"=0, "NAVX_OP_STATUS"=0, "YAW_STABLE"=FALSE, "Accel X"=0.0, "Accel Y"=0.0, "Accel Z"=0.0, "Accel Magnitude"=0.0, "Pitch Rate"=0.0, "Roll Rate"=0.0, "Yaw Rate"=0.0, "NavX Opened?"=FALSE}, "Tote Count"=0, "Have Trashcan"=FALSE, "Encoder Values"={"Left Encoder"={"Distance"=0.0, "Speed"=0.0, "Ticks"=0.0}, "Center Encoder"={"Distance"=0.0, "Speed"=0.0, "Ticks"=0.0}, "Right Encoder"={"Distance"=0.0, "Speed"=0.0, "Ticks"=0.0}}, "Power and Diagnostic Data"={"PDP Data"={"Battery Voltage"=0.0, "Temperature (degrees C)"=0.0, "Internal Battery R (Ohms)"=0.0, "Energy (J)"=0.0, "Power (W)"=0.0, "Total Current (A)"=0.0, "Battery Voltage Fault"=FALSE, "Temperature Fault"=FALSE, "Hardware Fault"=FALSE, "Currents"={"[0]"=0.0, "[1]"=0.0, "[2]"=0.0, "[3]"=0.0, "[4]"=0.0, "[5]"=0.0, "[6]"=0.0, "[7]"=0.0, "[8]"=0.0, "[9]"=0.0, "[10]"=0.0, "[11]"=0.0, "[12]"=0.0, "[13]"=0.0, "[14]"=0.0, "[15]"=0.0}, "Current Faults"={"[0]"=FALSE, "[1]"=FALSE, "[2]"=FALSE, "[3]"=FALSE, "[4]"=FALSE, "[5]"=FALSE, "[6]"=FALSE, "[7]"=FALSE, "[8]"=FALSE, "[9]"=FALSE, "[10]"=FALSE, "[11]"=FALSE, "[12]"=FALSE, "[13]"=FALSE, "[14]"=FALSE, "[15]"=FALSE}}, "PCM Data"={"Compressor Fault"=FALSE, "Solenoid Fault"=FALSE, "Compressor Enabled"=FALSE, "Hardware Fault"=FALSE, "Compressor Current"=0.0}, "roboRIO input voltage (V)"=0.0, "roboRIO input current (A)"=0.0, "3.3V Rail Short"=FALSE, "5 V Rail Short"=FALSE, "6 V Rail Short"=FALSE, "roboRIO Brownout"=FALSE, "Outputs Enabled?"=FALSE}, "Loop Timings"={"Roller Loop"=0, "Elevator Loop"=0, "US Loop"=0, "100ms Loop"=0, "Drivetrain Loop"=0}, "Ultrasonic Data"={"Left Distance"=0.0, "Right Distance"=0.0, "Center Distance"=0.0, "Left Distance Unfilter"=0.0, "Right Distance Unfilter"=0.0, "Center Distance Unfilter"=0.0}, "Zeroing Rollers?"=FALSE, "Drivetrain"={"Y (Throttle)"=0.0, "X (Steer)"=0.0, "Translation X"=0.0, "Center Wheel Down"=FALSE, "Mode"=enum."Manual", "Distance Drive finished?"=FALSE, "Y Target"=0.0, "X Target"=0.0, "Heading Target"=0.0, "Dist Drive Status"={"Y In Range"=FALSE, "X In Range"=FALSE, "Gyro In Range"=FALSE, "Y Dist"=0.0, "X Dist"=0.0, "Gyro"=0.0}, "Step Eject Lockout"=FALSE, "Gyro In Range?"=FALSE, "Yaw Comp Indicators"={"Rate Command"=0.0, "Rate Actual"=0.0, "Steer adjustment"=0.0}}, "Current Auto Command Data"={"Step ID"=0, "Command Type"=0, "Drive X"=0.0, "Drive Y"=0.0, "Heading"=0.0, "Max Exec. Time"=0, "Jump Type"=0, "Jump To"=0, "Jump Condition"=0, "Async Drive?"=0, "Roller Mode"=0, "Roller Align"=0, "Roller Closed?"=0, "Wait Condition"=0, "Elevator Mode"=0, "Elevator Command"=0, "Roller State"=0, "Hold Low?"=0, "Num Totes"=0, "Num Cans"=0.0, "Past Distance"=0.0, "Store Can?"=0.0, "X Speed"=0.0, "Y Speed"=0.0, "Yaw Angle Set"=0.0, "Grab Can"=0.0, "Roller Overide Speed"=0.0, "Force Load?"=0.0, "Set Idle"=0.0, "Eject"=0.0, "Pike Action"=0.0}, "Can Grabber"=FALSE, "Pike"={"Motor Out"=0.0, "Current"=0.0, "Limit Switch"=FALSE, "Current Limit"=FALSE, "State"=enum."Going Up", "Command"=enum."Auto Up"}} ("DB Disp Data"), binary string=w125) -> (value=w108:T53, error out=w124:errorcluster)  [unwired: 3 in, 1 out]
        n16 = call <vilib>:"Clear Errors.vi"("error in (no error)"=w124) -> ()  [unwired: 5 in, 2 out]
        n17 = Unbundle By Name(w108) -> ("Pike"=w66:T14, "Current Auto Command Data"=→"Current Auto Command Data":T17, "Drivetrain"=→"Drivetrain" →"Drivetrain 4":T18, "IMU Data"=w113:T38, "Pressure"=w96:dbl, "Pressure Transducer V"=→"Transducer Voltage":dbl, "Gyro Angle"=→"Gyro":dbl, "Power and Diagnostic Data"=→"Power and Diagnostic Data":T29, "Autonomous"=w109:T54, "Roller State Indicators"=w78:T44, "Encoder Values"=→"Encoder Values":T41, "Elevator Status Data"=w70:T10, "Zeroing Rollers?"=→"Zeroing Rollers?":bool)
        "Pressure" <- w96
        "Roller State Indicators" <- w78
        "Pressure 2" <- w96
        "IMU Data" <- w113
        "Elevator Status Data 2" <- w70
        "Elevator Status Data 3" <- w70
        "Pike Indicators" <- w66
        n18 = Unbundle By Name(w108) -> ("Tote Count"=→"Tote Count":i8, "Have Trashcan"=→"Trashcan? 2" →"Trashcan?":bool, "Loop Timings"=→"Loop Timings":T36, "Ultrasonic Data"=→"Ultrasonic Data" →"Ultrasonic Data 2" →"Ultrasonic Data 3":T9)
        n19 = Unbundle By Name(w109) -> ("Selected File"=→"Current File" →"Auton File":string, "Directory"=→"Directory":string, "Auton File Index"=→"File Index":i32, "Auton File Count"=→"Auton File Count":i32)
        n20 = Unbundle By Name(w113) -> ("NAVX_CAL_STATUS"=→"NAVX_CAL_STATUS":T3, "Roll"=→"Roll":sgl, "Pitch"=→"Pitch":sgl, "Yaw"=→"IMU Gyro":sgl)
        n21 = Unbundle By Name(w66) -> ("State"=w65:T15)
        n22 = case shown="\"Up\", Default" w65 {
          tunnel: [FALSE TRUE] -> w64
          frame "Up", Default {
          }
          frame "Down", "Going Down" {
          }
        }
        "Pike" <- w64
        n23 = Unbundle By Name(w70) -> ("Mode"=w84:T11, "Finger"=→"Finger":bool, "Stabilizer"=→"Stabilizer":bool)
        n24 = Unbundle By Name(w78) -> ("Roller Mode"=w77:T6)
        n25 = Unbundle By Name(w78) -> ("Roller Safety Open"=w72:bool, "Rollers Closed?"=w103:bool, "Zero Complete?"=w63:bool, "Roller Mode"=w101:T6, "Auto Roller State"=w100:T7, "Intake State"=w99:T8)
        n26 = case shown="\"Auto\"" w84 {
          tunnel: [u32 16711680 u32 16772394 u32 6618880] -> w87
          tunnel: ["MANUAL" "SAFE" "AUTO"] -> w79
          frame "Manual", Default {
          }
          frame "Safe" {
          }
          frame "Auto" {
          }
        }
        n27 = case shown="\"Auto\"" w77 {
          tunnel: [u32 16711680 u32 16772394 u32 6618880] -> w82
          tunnel: ["MANUAL" "SAFE" "AUTO"] -> w80
          frame "Manual", Default {
          }
          frame "Safe" {
          }
          frame "Auto" {
          }
        }
        n28 = Greater Or Equal?(x=w96, y=70.0) -> (x >= y?=w94:bool)
        n29 = Greater Or Equal?(x=w96, y=50.0) -> (x >= y?=w91:bool)
        n30 = Select(t=u32 16772394, s=w91, f=u32 16711680) -> (s? t:f=w92:u32)
        n31 = Bundle By Name(cluster=T5 {"Rollers Closed?"=FALSE, "Zero Complete?"=FALSE, "Roller Mode"=enum."Manual", "Auto Roller State"=enum."Grab Tote", "Intake State"=enum."Acquire Tote", "Left Out"=0.0, "Roller Safety Open"=FALSE, "Right Out"=0.0} ("Roller Indicators Thin"), "Roller Safety Open"=w72, "Rollers Closed?"=w103, "Zero Complete?"=w63, "Roller Mode"=w101, "Auto Roller State"=w100, "Intake State"=w99) -> (→"Roller Indicators":T5)
        n32 = Select(t=u32 6618880, s=w94, f=w92) -> (s? t:f=w88:u32)
        n33 = Bundle(w87, w87) -> (w86:cluster{u32, u32})  [unwired: 1 in]
        n34 = Bundle(w82, w82) -> (w83:cluster{u32, u32})  [unwired: 1 in]
        n35 = property on="Pressure" class="DigNum (strict)"("NumText.BGColor"=w88) -> ()  [unwired: 2 in, 2 out]
        n36 = property on="Pressure 2" class="DigNum (strict)"("NumText.BGColor"=w88) -> ()  [unwired: 2 in, 2 out]
        n37 = Build Array(w86, w86) -> (w85:cluster{u32, u32}[])
        n38 = Build Array(w83, w83) -> (w81:cluster{u32, u32}[])
        n39 = property on="Elevator Mode" class="Bool (strict)"("BoolText.Text"=w79, "Colors [4]"=w85) -> ()  [unwired: 2 in, 2 out]
        n40 = property on="Roller Mode" class="Bool (strict)"("BoolText.Text"=w80, "Colors [4]"=w81) -> ()  [unwired: 2 in, 2 out]
        "Status Info" <- w128
        "Robot Metrics" <- w123
        "DS TCP" <- w127
        "Control Info" <- w122
      }
    }
  }
  n41 = vi-ref "Playback Controls.vi"() -> (w40:refnum<vi>)
  n42 = call "Initialize Camera and CheckList.vi"() -> ("Cluster"=w26:cluster{"value":i32, "value":i32, "index":i32}, "Array"=w25:cluster{string[]}[], "File Refnum"=w24:T55)  [unwired: 9 in]
  n43 = property class="Pnl"(reference=w41) -> ("Panes[]"=w42:refnum<vi>[])  [unwired: 1 in, 2 out]
  n44 = property on="Camera Settings" class="Clust (strict)"("Val(Sgnl)"=w26) -> ()  [unwired: 2 in, 2 out]
  n45 = Index Array(array=w42) -> (element=w23:refnum<vi>)  [unwired: 1 in]
  n46 = while {
    tunnel: w25 -> [w149]
    shift-right: [w148] -> _
    shift-left: w24 -> [w147]
    tunnel: [w146] -> _
    tunnel: w40 -> [w145]
    tunnel: w39 -> [w144]
    tunnel: w38 -> [_]
    tunnel: w35 -> [w143]
    i -> [w146]
    stop <- FALSE stop-if-true
    n47 = event shown="[2] \"Rec Mode\": Value Change" {
      selector: w144 -> [_ _ _ _ _ _]
      dyn-events: [_ _ w193 _ _ _] -> _
      timeout: _ -> [_ _ _ _ _ _]
      tunnel: w149 -> [w153 w183 _ _ _ _]
      tunnel: [w152 w176 w195 w209 w210 w220] -> w148
      tunnel: w147 -> [w151 w176 w195 w209 w210 w220]
      tunnel: w145 -> [_ _ w196 _ w213 _]
      tunnel: w143 -> [_ _ w191 _ _ _]
      event "DB Camera Config": Value Change {
        # "Show or hide the cluster of controls, store in ini file"
        n48 = event-data() -> ("NewVal"=w154:bool)  [unwired: 1 in]
        n49 = case shown="False" w154 {
          tunnel: w153 -> [w163 _]
          tunnel: [w156 w174] -> w152
          tunnel: w151 -> [w155 w174]
          frame False {
            w170 = "Camera"
            w173 = FALSE ("Visible")
            n50 = local read "Camera Settings"() -> (w162:T22)
            n51 = Index Array(array=w163) -> (element=w166:cluster{string[]})  [unwired: 1 in]
            n52 = Unbundle(w162) -> ("Frame Rate"=w161:i32, "Compression"=w160:i32, "Size"=w164:u16)
            n53 = Unbundle(w166) -> (w165:string[])
            n54 = Index Array(array=w165, index=w164) -> (element=w159:string)
            n55 = call-poly <vilib>:"Write Key.vi"("section"=w170, "value"=w159, "key"="Size", "refnum"=w155) -> ("refnum out"=w172:T55)  [unwired: 2 in, 5 out]
            n56 = call-poly <vilib>:"Write Key.vi"("section"=w170, "value"=w161, "key"="FrameRate", "refnum"=w172) -> ("refnum out"=w171:T55)  [unwired: 1 in, 6 out]
            n57 = property on="Camera Settings" class="Clust (strict)"("Visible"=w173) -> ()  [unwired: 2 in, 2 out]
            n58 = local write "DB Camera Config"(w173) -> ()
            n59 = call-poly <vilib>:"Write Key.vi"("section"=w170, "value"=w160, "key"="Compression", "refnum"=w171) -> ("refnum out"=w157:T55)  [unwired: 1 in, 6 out]
            n60 = call <vilib>:"Close Config Data.vi"("refnum"=w157) -> ("file path"=w158:path)  [unwired: 2 in, 8 out]
            n61 = call <vilib>:"Open Config Data.vi"("configuration file path"=w158) -> ("refnum"=w156:T55)  [unwired: 8 in, 2 out]
          }
          frame True {
            n62 = property on="Camera Settings" class="Clust (strict)"("Visible"=TRUE) -> ()  [unwired: 2 in, 2 out]
          }
        }
      }
      event "Camera Settings": Value Change {
        # "Update summary string when any elements of DB camera change"
        n63 = event-data() -> ("NewVal"=w187:T22)  [unwired: 1 in]
        n64 = Index Array(array=w183) -> (element=w182:cluster{string[]})  [unwired: 1 in]
        n65 = Unbundle(w187) -> ("Frame Rate"=w178:i32, "Compression"=w177:i32, "Size"=w180:u16)
        n66 = Unbundle(w182) -> (w181:string[])
        n67 = Index Array(array=w181, index=w180) -> (element=w179:string)
        n68 = Format Into String(format string="%s   %dfps   %d%%", w179, w178, w177) -> (resulting string=w184:string)  [unwired: 2 in, 1 out]
        n69 = Build Array(w184) -> (w185:string[])
        n70 = property on="DB Camera Config" class="Bool (strict)"("Strings [4]"=w185) -> ()  [unwired: 2 in, 2 out]
      }
      event "Rec Mode": Value Change {
        # "Update globals for recording mode and path to read log from.\nClear when logging and let NetworkTables set path for vision to\nuse."
        n71 = event-data() -> ("NewVal"=w197:enum32{"Stop", "Record", "Playback"})  [unwired: 1 in]
        n72 = global write "WPI_DashboardLogging Global.vi" "Logging Filename"(path "") -> ()
        n73 = case shown="\"Playback\"" w197 {
          tunnel: w196 -> [_ w199 w203]
          tunnel: [_ _ w207] -> w193
          tunnel: [_ _ w206] -> _
          tunnel: w191 -> [_ _ w201]
          tunnel: cluster{i32, i32} {-250, 170} -> [_ _ w200]
          tunnel: [_ _ T56 {"Image Size"=TRUE, "Image Type"=TRUE, "Pixel Value"=TRUE, "ROI Information"=TRUE, "Zoom Factor"=FALSE} ("Image Information Shown:All Elements")] -> w189
          tunnel: [_ _ TRUE ("Zoom Factor")] -> w188
          frame Default {
          }
          frame "Stop", "Record" {
            # "Place Window too"
            n74 = invoke class="VI" method="FP.Close"(reference=w199) -> (reference out=w198:refnum<vi>)  [unwired: 2 in, 2 out]
            n75 = invoke class="VI" method="Abort VI"(reference=w198) -> ()  [unwired: 2 in, 3 out]
          }
          frame "Playback" {
            n76 = call "Open Playback Panel.vi"("Offset"=w200, "DB VI Ref"=w201, "Playback in"=w203) -> ("Playback out"=w202:refnum<vi>)  [unwired: 8 in]
            n77 = register-events(w202) -> (reference out=w207:refnum<event-registration>, error out=w206:errorcluster)  [unwired: 2 in]
          }
        }
        n78 = global write "WPI_DashboardLogging Global.vi" "Recording"(w197) -> ()
        n79 = property on="Axis Display" class="ImageControl"("Image Information Shown"=w189, "Image Information Visible"=w188) -> ()  [unwired: 2 in, 2 out]
        n80 = call <vilib>:"WPI_DashboardNT Log FieldName Cache.vi"("Operation"=enum16{"Lookup/Add", "Index", "Clear"}."Clear") -> ()  [unwired: 8 in, 3 out]
      }
      event Panel Close {
        w208 = enum32{"Stop", "Record", "Playback"}."Stop" ("Rec Mode")
        # "Playback window has been closed, abort"
        n81 = event-data() -> ()  [unwired: 1 in, 4 out]
        n82 = local write "Rec Mode"(w208) -> ()
        n83 = global write "WPI_DashboardLogging Global.vi" "Recording"(w208) -> ()
      }
      event Panel Close {
        # "Abort playback window and ourself"
        n84 = event-data() -> ()  [unwired: 1 in, 4 out]
        n85 = invoke class="VI" method="FP.Close"(reference=w213) -> (reference out=w212:refnum<vi>)  [unwired: 2 in, 2 out]
        n86 = invoke class="VI" method="Abort VI"(reference=w212) -> (error out=w211:errorcluster)  [unwired: 2 in, 2 out]
        n87 = invoke class="VI" method="Abort VI"(error in=w211) -> ()  [unwired: 2 in, 3 out]
      }
      event "Vision": Value Change {
        # "Enable/Disable Compression slider.\nHW USB is hard-coded into the camera"
        n88 = event-data() -> ("NewVal"=w219:u16)  [unwired: 1 in]
        n89 = Equal?(x=w219, y=u32 2 ("milliseconds to wait")) -> (x = y?=w217:bool)
        n90 = Select(t=T57."Disabled and Grayed Out" ("Disabled"), s=w217, f=T57."Enabled" ("Disabled")) -> (s? t:f=w214:T57)
        n91 = property on="Compression" class="Slide (strict)"("DisabledEnum"=w214) -> ()  [unwired: 2 in, 2 out]
      }
    }
  }
  n92 = while {
    tunnel: w23 -> [w222]
    i -> [w225]
    stop <- FALSE stop-if-true
    n93 = Wait (ms)(milliseconds to wait=u32 100) -> ()  [unwired: 1 out]
    n94 = case shown="\"Playback\"" "Rec Mode" {
      tunnel: w225 -> [_ _ w240]
      tunnel: [u32 1973790 ("Base Color") u32 11141120 ("Target Color") w232] -> w221
      frame "Stop", Default {
        # "Reset the color, extra updates don't cost much"
      }
      frame "Record" {
      }
      frame "Playback" {
        # "Playback"
        n95 = Quotient & Remainder(x=w240, y=u32 50 ("milliseconds to wait")) -> (x-y*floor(x/y)=w236:u32)  [unwired: 1 out]
        n96 = Divide(x=w236, y=u32 50 ("milliseconds to wait")) -> (x/y=w233:dbl)
        n97 = Multiply(x=6.283185307179586, y=w233) -> (x*y=w238:dbl)
        n98 = Sine(x=w238) -> (sin(x)=w237:dbl)
        n99 = Absolute Value(x=w237) -> (abs(x)=w231:dbl)
        n100 = call "Interpolate RGB Color.vi"("Proportion"=w231, "Target Color"=u32 30976, "Base Color"=u32 2829099) -> ("Result Color"=w232:u32)  [unwired: 8 in]
      }
    }
    n101 = property class="Pane"(reference=w222, "PaneColor"=w221) -> ()  [unwired: 1 in, 2 out]
  }
  n102 = property class="Pane"(reference=w23, "Origin"=T52 {"Horizontal"=-1561, "Vertical"=-62}) -> ()  [unwired: 1 in, 2 out]
  n103 = while {
    tunnel: u16 1741 ("timeout ms (25000)") -> [w244]
    stop <- FALSE stop-if-true
    n104 = TCP Create Listener(10:w244) -> (0:w241:errorcluster, 3:w243:refnum<k5>)  [unwired: 4 in, 1 out]
    n105 = case shown="No Error" w241 {
      tunnel: w243 -> [w245 _]
      frame No Error {
        # "Loop 7. Wait for DS connections"
        n106 = while {
          tunnel: w245 -> [w248]
          stop <- FALSE stop-if-true
          n107 = TCP Wait On Listener(11:w248) -> (0:w246:errorcluster, 4:w247:refnum<k5>)  [unwired: 3 in, 3 out]
          n108 = local write "TCP"(w247) -> ()
          n109 = case shown="Error" w246 {
            frame No Error {
            }
            frame Error {
              n110 = Wait (ms)(milliseconds to wait=u32 100) -> ()  [unwired: 1 out]
            }
          }
        }
      }
      frame Error {
      }
    }
  }
  n111 = property on="Camera Settings" class="Clust (strict)"("Visible"=w34) -> ()  [unwired: 2 in, 2 out]
  n112 = local write "DB Camera Config"(w34) -> ()
  n113 = call <vilib>:"Intialize Keyboard.vi"() -> ("device ID"=w5:refnum<k1>)  [unwired: 10 in, 1 out]
  n114 = while {
    tunnel: w5 -> [w253]
    stop <- FALSE stop-if-true
    # "(Keyboard: UDP 5803)"
    # "Send the keyboard to the robot every 50 ms"
    n115 = call-poly <vilib>:"Acquire Input Data.vi"("device ID"=w253) -> ("keys pressed"=w252:T58)  [unwired: 16 in, 2 out]
    n116 = local read "Robot IP"() -> (w251:string)
    n117 = call "Send Keyboard Data.vi"("Robot IP"=w251, "keys pressed"=w252) -> ()  [unwired: 10 in]
    n118 = Wait (ms)(milliseconds to wait=u32 50) -> ()  [unwired: 1 out]
  }
  n119 = global write "WPI_DashboardLogging Global.vi" "Recording"(w36) -> ()
  n120 = local write "Rec Mode"(w36) -> ()
  n121 = Generate Occurrence() -> (w4:refnum<k4>)
  n122 = while {
    tunnel: w48 -> [w263]
    tunnel: w47 -> [_]
    tunnel: w4 -> [w257]
    tunnel: w1 -> [w256]
    stop <- FALSE stop-if-true
    # "Axis cam"
    n123 = case shown="False" "Use File" {
      tunnel: w263 -> [w274 w282]
      tunnel: [w273 w281] -> w262
      tunnel: [w272 w275] -> w261
      tunnel: [w271 62.4 ("FPS")] -> w260
      tunnel: [w270 6.24 ("Bandwidth (Mbps)")] -> w259
      frame False {
        # "Optionally read the DB image,\nlog, or retrieve images from a\nlogged match"
        n124 = local read "Rec Mode"() -> (w268:enum32{"Stop", "Record", "Playback"})
        n125 = call "624WPI_CameraRead MJPG for Dashboard.vi"("Camera Settings"="Camera Settings", "USB Cam TCP Port"=u16 5800, "Rec Mode"=w268, "Camera IP"="axis-camera.local", "Camera Mode"="Camera Mode", "Refnum in"=w274) -> ("Active"=w272:bool, "Refnum out"=w273:T1, "FPS"=w271:dbl, "Bandwidth (Mbps)"=w270:dbl)  [unwired: 2 in]
      }
      frame True {
        n126 = call "IMAQ ReadFile"("File Path"="File Path", "Image"=w282) -> ("error out"=w277:errorcluster, "Image Out"=w281:T1)  [unwired: 5 in, 3 out]
        n127 = Unbundle By Name(w277) -> ("status"=w276:bool)
        n128 = Not(x=w276) -> (.not. x?=w275:bool)
      }
    }
    n129 = case shown="True" w261 {
      tunnel: w262 -> [_ w293]
      tunnel: w259 -> [_ w292]
      tunnel: w260 -> [_ w291]
      tunnel: w257 -> [_ w290]
      tunnel: w256 -> [_ w284]
      frame False {
        # "Sleep for 500ms"
        n130 = Wait Until Next ms Multiple(millisecond multiple=u32 500) -> ()  [unwired: 1 out]
      }
      frame True {
        # "Update Mbps LED"
        n131 = call "IMAQ Clear Overlay"("Image"=w293) -> ("error out"=w297:errorcluster, "Image Out"=w287:T1)  [unwired: 2 in, 7 out]
        n132 = case shown="4, 5" w292 {
          tunnel: [u32 6618880 ("Color Box") u32 16776722 ("Color Box") u32 16716800 ("Color Box")] -> w294
          frame Default {
          }
          frame 4, 5 {
          }
          frame 6.. {
          }
        }
        n133 = Unbundle By Name(w297) -> ("status"=w298:bool)
        n134 = Bundle("Color Box"=w294, "Color Box"=w294) -> (w296:cluster{"Color Box":u32, "Color Box":u32})  [unwired: 1 out]
        n135 = property on="Image Message" class="Str"("Visible"=w298) -> ()  [unwired: 2 in, 2 out]
        n136 = Build Array(w296) -> (w295:cluster{"Color Box":u32, "Color Box":u32}[])
        n137 = disable-structure shown="Enabled" {
          disable-tunnel: [w307 _] -> _
          disable-tunnel: [w306 _] -> _
          disable-tunnel: [w303 w312] -> w289
          disable-tunnel: w287 -> [w300 w314]
          disable-tunnel: [w299 w311] -> w285
          disable-tunnel: w284 -> [_ w310]
          frame Disabled {
            n138 = call "624 Detect Retroreflective Vision Totes.vi"("Limit %"="Min target size %", "Filter Settings"="Filter Settings", "Ring Light Color"="Ring Light Color", "Image Src"=w300, "Camera FOV width"="Camera FOV width") -> ("Detected totes"=w307:T27[], "Masked"=w304:T1, "Processed Img"=w299:T1)  [unwired: 4 in]
            "Detected totes" <- w307
            n139 = local read "Robot IP"() -> (w306:string)
            n140 = Select(t=w304, s="Mask View", f=w299) -> (s? t:f=w303:T1)
          }
          frame Enabled {
            n141 = call "Draw Feeder Overlay.vi"("Rectangle"="Rectangle", "Refnum in"=w314) -> ("Refnum out"=w312:T1)  [unwired: 9 in]
            n142 = call "IMAQ Copy"("Image Dst"=w310, "Image Src"=w312) -> ("Image Dst Out"=w311:T1)  [unwired: 4 in, 1 out]
          }
        }
        "Axis Display" <- w289
        "Axis Cam" <- w285
        n143 = property on="Mbps 2" class="Bool (strict)"("Colors [4]"=w295) -> ()  [unwired: 2 in, 2 out]
        n144 = control-ref of="Axis Display"() -> (w288:refnum<vi>)
        n145 = control-ref of="Ring Light Color"() -> (w286:refnum<vi>)
        n146 = call "Calibration Helper.vi"("Color Display"=w286, "Image"=w287, "Image Ctl Refnum"=w288) -> ()  [unwired: 8 in, 1 out]
        n147 = Set Occurrence(w290) -> ()
        "Mbps" <- w292
        "fps" <- w291
      }
    }
  }
  n148 = while {
    tunnel: w15 -> [w329]
    tunnel: w4 -> [w318]
    stop <- FALSE stop-if-true
    # "USB Cam here"
    n149 = local read "Camera IP"() -> (w328:string)
    n150 = local read "Rec Mode"() -> (w326:enum32{"Stop", "Record", "Playback"})
    n151 = call "624WPI_CameraRead MJPG for Dashboard.vi"("Camera Settings"="Camera Settings 2", "USB Cam TCP Port"=u16 1180, "Rec Mode"=w326, "Camera IP"=w328, "Camera Mode"="Vision", "Refnum in"=w329) -> ("Active"=w324:bool, "Refnum out"=w323:T1, "FPS"=w320:dbl, "Bandwidth (Mbps)"=w322:dbl)  [unwired: 2 in]
    n152 = case shown="True" w324 {
      tunnel: w323 -> [_ w332]
      tunnel: w322 -> [_ w334]
      tunnel: w320 -> [_ w333]
      tunnel: w318 -> [_ w331]
      frame False {
        n153 = Wait Until Next ms Multiple(millisecond multiple=u32 500) -> ()  [unwired: 1 out]
      }
      frame True {
        n154 = Set Occurrence(w331) -> ()
        "USB Cam" <- w332
        "Mbps 2" <- w334
        "fps 2" <- w333
      }
    }
  }
  n155 = UDP Open(11:u16 0 ("port")) -> (port=w29:refnum<k16>)  [unwired: 4 in, 2 out]
  n156 = while {
    tunnel: w29 -> [w355]
    stop <- FALSE stop-if-true
    # "Send control parameters to robot 4x per second on UDP port 5801"
    n157 = Unbundle By Name("Elevator") -> ("Presets.HP Load Drop"=w337:dbl)
    n158 = Select(t=0.0, s="Dallas load", f=w337) -> (s? t:f=w336:dbl)
    n159 = Wait (ms)(milliseconds to wait=u32 250) -> ()  [unwired: 1 out]
    n160 = Bundle By Name(cluster="Elevator", "Presets.HP Load Drop"=w336) -> (w339:T48)
    n161 = Bundle By Name(cluster=T59 {"Cam Exposure"=0.0, "Go to angle"=0.0, "Steer PID Gains"={"proportional gain (Kc)"=1.0, "integral time (Ti, min)"=0.01, "derivative time (Td, min)"=0.0}, "Steer PID output Range"={"output high"=1.0, "output low"=-1.0}, "Pressure m \nValue"=0.0, "Pressure b \nValue"=0.0, "Roller Command Cluster "={"Intake Speed"=0.0, "Turn In Speed"=0.0, "Unload Speed"=0.0, "Turn Out Speed"=0.0, "Ping Align Tolerance"=1000.0, "Tote Range Threshold"=0.0, "Right Pot 0"=0.0, "Pot Threshold"=0.0, "Left Pot 0"=0.0, "Manual 0s?"=FALSE, "Right Pot Scale"=0.0, "Left Pot Scale"=0.0, "0 wait time"=0, "Zero Pots"=FALSE, "Min Elevator Height"=0.0, "Eject Time"=0.0, "Eject US Threshold"=0.0, "Anti-Twitch Time"=0, "Ping Caring Threshold"=0.0, "Pot Diff Threshold"=0.0, "Pinch Sustain"=0, "Absorb Give Up Threshold"=0.0, "Untip In Threshold"=0.0, "Untip Grab Range"=0.0, "Ultrasonic Hold Time"=0, "Landscape Absorb Time"=0, "Pot Use Wait Time"=0, "Can Turn Stop Range"=0.0, "Ignore Pressure"=FALSE, "HP Load Speed"=0.0}, "Elevator"={"PID Output Range"={"output high"=100.0, "output low"=-100.0}, "PID gains"={"proportional gain (Kc)"=1.0, "integral time (Ti, min)"=0.01, "derivative time (Td, min)"=0.0}, "Height Tolerance"=0.0, " Encoder Constant"=0.0, "Safe Mode Max Speed"=0.0, "Eject Time"=0.0, "Zeroing Speed"=0.0, "Presets"={"Pickup 2 w/ Tote"=0.0, "Pickup 2 w/ Trashcan"=0.0, "Pickup 3 w/ Tote"=0.0, "Pickup 3 w/ Trashcan"=0.0, "Bottom"=0.0, "Pickup 1 w/ Tote"=0.0, "Pickup Trashcan"=0.0, "Pickup 1 w/ Trashcan"=0.0, "Eject"=0.0, "Hold Low"=0.0, "Step add height"=0.0, "Untip Lift"=0.0, "Drop Stack"=0.0, "HP Load Hold"=0.0, "HP Load Drop"=0.0, "HP Load Finger"=0.0, "HP Load Hold Can"=0.0, "Store can max"=0.0, "HP Drag Score"=0.0, "HP Store can max"=0.0, "HP Drag Finish"=0.0, "HP Carry min"=0.0, "HP Finger Anti-Crash"=0.0, "Finger trashcan avoid"=0.0}, "Ping Detect Threshold"=0.0, "Trashcan Detect Threshold"=0.0, "Zero Filter Time"=0.0, "Stabilizer Open Time"=0.0, "Zero Creep Speed"=0.0, "Max Current"=0.0, "Current Trip Time"=0.0, "Abort Pitch"=0.0, "Finger m"=0.0, "Finger b"=0.0, "Finger max "=0.0, "Finger Stabilizer"=0.0, "Finger Store"=0.0, "Finger Stop Store"=0.0, "Stabilizer Close Time"=0.0, "HP Finger Store"=0.0, "HP Finger Stop Store"=0.0, "Finger min"=0.0, "Unstick gain"=0.0, "Roller Wait"=0.0}, "Encoder Control"={"Left Tick Constant"=1.0, "Right Tick Constant"=0.0, "Center Tick Constant"=0.0, "Reset?"=FALSE, "Y Dist"={"PID gains"={"proportional gain (Kc)"=1.0, "integral time (Ti, min)"=0.0, "derivative time (Td, min)"=0.0}}, "X Dist"={"PID gains"={"proportional gain (Kc)"=1.0, "integral time (Ti, min)"=0.0, "derivative time (Td, min)"=0.0}}, "Y Stop Thresh"=0.0, "Y Stop Speed"=0.0, "X Stop Thresh"=0.0, "X Stop Speed"=0.0}, "Auton Settings"={"Drive Dist Window Size"=0.0}, "Drivetrain Settings"={"Gyro Tolerance"=0.0, "Strafe Correct max steer"=0.4, "Strafe Timer Wait"=250.0, "Throttle Ramp (ms)"=0.0, "Strafe Ramp (ms)"=0.0, "Angular rate compensation"=FALSE, "Throttle to Rate Scale"=0.0, "Rate compensation gain"=0.0, "Creep Steer"=0.0, "Creep Throttle"=0.0}, "Lance"={"Down Speed"=0.0, "Up Speed"=0.0, "Max Down Time"=0.0, "Max Up Time"=0.0, "Current Limit"=0.0}} ("DB Control Data"), "Cam Exposure"="Cam Exposure", "Go to angle"="Go to angle", "Steer PID Gains"="Yaw PID Gains", "Steer PID output Range"="Yaw PID Output Range", "Pressure m \nValue"="Pressure m Value", "Pressure b \nValue"="Pressure b Value", "Roller Command Cluster"="Roller Settings", "Elevator"=w339, "Encoder Control"="Encoder Control", "Drivetrain Settings"="Drivetrain Settings") -> (w351:T59)
    n162 = local read "Robot IP"() -> (w352:string)
    n163 = Empty String/Path?(string/path=w352) -> (empty?=w353:bool)
    n164 = case shown="False" w353 {
      tunnel: w355 -> [w363 _]
      tunnel: w351 -> [w359 _]
      tunnel: w352 -> [w357 _]
      frame False {
        n165 = Flatten To String(anything=w359) -> (data string=w361:string, error out=w360:errorcluster)  [unwired: 3 in, 1 out]
        n166 = String To IP(1:w357) -> (0:w358:u32)
        n167 = UDP Write(address=w358, port or service name=u16 5801, connection ID=w363, data in=w361, 8:w360) -> ()  [unwired: 1 in, 2 out]
      }
      frame True {
        # "The robot IP is not\nready yet, don't try\nto send data"
      }
    }
  }
  n168 = vi-ref "Image Display.vi"() -> (w7:refnum<vi>)
  n169 = while {
    tunnel: w4 -> [w367]
    stop <- FALSE stop-if-true
    n170 = local read "Mbps"() -> (w366:dbl)
    n171 = local read "Mbps 2"() -> (w365:dbl)
    n172 = Wait on Occurrence(2:w367) -> ()  [unwired: 2 in, 1 out]
    n173 = Add(x=w366, y=w365) -> (x+y=→"Total mbps":dbl)
    n174 = local read "USB Cam"() -> (w369:T1)
    n175 = local read "Axis Cam"() -> (w368:T1)
    n176 = call "Image Display.vi"("Img In 2"=w369, "Img In"=w368) -> ()  [unwired: 10 in]
  }
  n177 = control-ref of="Dashboard Tab"() -> (w11:refnum<vi>)
  n178 = invoke class="VI" method="FP.Open"(reference=w7, "Activate"=TRUE ("Activate?"), "State"=T51."Standard") -> (reference out=w10:refnum<vi>)  [unwired: 2 in, 4 out]
  n179 = while {
    stop <- FALSE stop-if-true
    # "Clear the background of the message\nbox after a while"
    n180 = event shown="[0] \"DumbDash Message\": Value Change" {
      selector: _ -> [_]
      dyn-events: _ -> [_]
      timeout: _ -> [_]
      event "DumbDash Message": Value Change {
        n181 = event-data() -> ()  [unwired: 1 in, 3 out]
        n182 = flat-sequence {
          frame #0 {
            n183 = Wait (ms)(milliseconds to wait=u32 3000) -> ()  [unwired: 1 out]
          }
          frame #1 {
            w374 = u32 3552822
            n184 = property on="DumbDash Message" class="Str"("Text.BGColor"=w374, "Text.BG Color"=w374, "Blinking"=FALSE) -> ()  [unwired: 2 in, 2 out]
          }
        }
      }
    }
  }
  n185 = call "DumbDash Load Controls.vi"("TabControl in"=w11) -> ("Array"=w14:T61[])  [unwired: 10 in]
  n186 = property class="VI"(reference=w10, "Front Panel.ShowMenuBar"=w6, "TB.Visible"=w6, "Front Panel.Resizeable"=w6) -> ()  [unwired: 1 in, 2 out]
  n187 = call <vilib>:"Read PNG File.vi"("path to PNG file"=path "tote_stack_pics/gray_tote.png" ("path to JPEG file")) -> ("image data"=w20:T63)  [unwired: 8 in, 2 out]
  n188 = control-ref of="DumbDash Message"() -> (w13:refnum<vi>)
  n189 = while {
    tunnel: w14 -> [w386]
    tunnel: w13 -> [w385]
    stop <- FALSE stop-if-true
    n190 = local read "Robot IP"() -> (w379:string)
    n191 = local read "Camera IP"() -> (w383:string)
    n192 = local read "Robot IP"() -> (w384:string)
    n193 = Equal?(x=w379, y="0.0.0.0") -> (x = y?=w377:bool)
    n194 = Empty String/Path?(string/path=w383) -> (empty?=w381:bool)
    n195 = Empty String/Path?(string/path=w384) -> (empty?=w382:bool)
    n196 = case shown="True" "Save" {
      tunnel: w386 -> [_ w402]
      tunnel: w385 -> [_ w401]
      frame False {
      }
      frame True {
        n197 = flat-sequence {
          tunnel: w402 -> [w404]
          tunnel: w401 -> [w403]
          frame #0 {
            n198 = call "DumbDash Save Values.vi"("Message Box"=w403, "Controls In"=w404) -> ()  [unwired: 10 in]
          }
          frame #1 {
            n199 = local write "Save"(FALSE ("Save")) -> ()
          }
        }
      }
    }
    n200 = case shown="True" "Load" {
      tunnel: w386 -> [_ w397]
      tunnel: w385 -> [_ w396]
      frame False {
      }
      frame True {
        n201 = flat-sequence {
          tunnel: w397 -> [w399]
          tunnel: w396 -> [w398]
          frame #0 {
            n202 = call "DumbDash Load Values.vi"("Message Box"=w398, "Controls In"=w399) -> ()  [unwired: 10 in]
          }
          frame #1 {
            n203 = local write "Load"(FALSE ("Load")) -> ()
          }
        }
      }
    }
    n204 = Compound Arithmetic op=OR(w377, w382, w381) -> (w380:bool)
    n205 = case shown="True" w380 {
      frame False {
        n206 = property on="DumbDash Message" class="Str"("Blinking"=FALSE) -> ()  [unwired: 2 in, 2 out]
      }
      frame True {
        n207 = disable-structure shown="Disabled" {
          frame Disabled {
            w395 = u32 16711680
            n208 = property on="DumbDash Message" class="Str"("Blinking"=TRUE, "Text.BGColor"=w395, "Text.BG Color"=w395) -> ()  [unwired: 2 in, 2 out]
            "DumbDash Message" <- "Restart the Driver Station!! Bad IP" ("DumbDash Message")
          }
          frame Enabled {
          }
        }
      }
    }
    n209 = disable-structure shown="RUN_TIME_ENGINE==True" {
      disable-tunnel: "stop" -> [w390 w391]
      frame condition #0 {
        # "Close the build DB"
        n210 = Quit LabVIEW(quit? (T)=w390) -> ()
      }
      frame condition #1 (active) {
        n211 = Stop(stop? (T)=w391) -> ()
      }
    }
    n212 = Wait (ms)(milliseconds to wait=u32 250) -> ()  [unwired: 1 out]
  }
  n213 = local write "Load"(TRUE ("Load")) -> ()
  n214 = call <vilib>:"Read PNG File.vi"("path to PNG file"=path "tote_stack_pics/bin.png" ("path to JPEG file")) -> ("image data"=w18:T63)  [unwired: 8 in, 2 out]
  n215 = while {
    tunnel: w20 -> [w421]
    tunnel: w18 -> [w420]
    stop <- FALSE stop-if-true
    n216 = local read "Robot Mode"() -> (w409:T4)
    n217 = local read "IMU Data"() -> (w417:T38)
    n218 = Unbundle By Name(w417) -> ("Data Valid?"=w413:bool)
    n219 = Equal?(x=w409, y=T4."Disconnected") -> (x = y?=w406:bool)
    n220 = Equal?(x=w409, y=T4."No Code") -> (x = y?=w407:bool)
    n221 = Or(x=w406, y=w407) -> (x .or. y?=w408:bool)
    n222 = Wait (ms)(milliseconds to wait=u32 50) -> ()  [unwired: 1 out]
    n223 = Or(x=w413, y=w408) -> (x .or. y?=w412:bool)
    n224 = case shown="False" w412 {
      tunnel: [w431 u32 2829099 ("Base Color")] -> w414
      frame False {
        n225 = Tick Count (ms)() -> (millisecond timer value=w432:u32)
        n226 = Quotient & Remainder(x=w432, y=u32 1000 ("milliseconds to wait")) -> (x-y*floor(x/y)=w439:u32)  [unwired: 1 out]
        n227 = Divide(x=w439, y=u32 1000 ("milliseconds to wait")) -> (x/y=w436:dbl)
        n228 = Multiply(x=6.283185307179586, y=w436) -> (x*y=w441:dbl)
        n229 = Sine(x=w441) -> (sin(x)=w440:dbl)
        n230 = Absolute Value(x=w440) -> (abs(x)=w435:dbl)
        n231 = call "Interpolate RGB Color.vi"("Proportion"=w435, "Target Color"=u32 16711680, "Base Color"=u32 2829099) -> ("Result Color"=w431:u32)  [unwired: 8 in]
      }
      frame True {
      }
    }
    n232 = local read "Tote Count"() -> (w419:i32)
    n233 = while {
      tunnel: w419 -> [w454]
      shift-right: [w455] -> w423
      shift-left: cluster{"x":i16, "y":i16} {"x"=0, "y"=0} ("top left point(0, 0)") -> [w465]
      shift-right: [w462] -> _
      shift-left: w421 -> [w462]
      shift-right: [w461] -> _
      shift-left: 0 -> [w460]
      shift-right: [w463] -> w426
      shift-left: picture data[5B] ("new picture") -> [w459]
      tunnel: [w454] -> w425
      stop <- w467 stop-if-true
      n234 = Multiply(x=-54, y=w460) -> (x*y=w458:i32)
      n235 = call <vilib>:"Unflatten Pixmap.vi"("image data"=w462) -> ("24-bit pixmap"=w466:u32[][])  [unwired: 4 in, 6 out]
      n236 = Add(x=w458, y=440) -> (x+y=w456:i32)
      n237 = Bundle By Name(cluster=w465, "y"=w456) -> (w455:cluster{"x":i16, "y":i16})
      n238 = Increment(x=w460) -> (x+1=w461:i32)
      n239 = call-poly <vilib>:"Draw Unflattened Pixmap.vi"("picture"=w459, "top left point(0, 0)"=w455, "data (RGB format)"=w466) -> ("new picture"=w463:picture)  [unwired: 6 in]
      n240 = Greater?(x=w461, y=w454) -> (0:w467:bool)
    }
    n241 = local read "Trashcan?"() -> (w418:bool)
    n242 = property on="Gyro" class="Knob (strict)"("BGColor"=w414) -> ("DigDisps[]"=w416:refnum<vi>[])  [unwired: 2 in, 2 out]
    n243 = case shown="True" w418 {
      tunnel: w426 -> [w444 w451]
      tunnel: w425 -> [_ _]
      tunnel: w420 -> [_ w453]
      tunnel: [w444 w450] -> w424
      tunnel: w423 -> [_ w447]
      frame False {
      }
      frame True {
        n244 = Unbundle By Name(w447) -> ("y"=w449:i16)
        n245 = call <vilib>:"Unflatten Pixmap.vi"("image data"=w453) -> ("24-bit pixmap"=w452:u32[][])  [unwired: 4 in, 6 out]
        n246 = Subtract(x=w449, y=i16 101) -> (x-y=w446:i16)
        n247 = Bundle By Name(cluster=w447, "y"=w446) -> (w445:cluster{"x":i16, "y":i16})
        n248 = call-poly <vilib>:"Draw Unflattened Pixmap.vi"("picture"=w451, "top left point(0, 0)"=w445, "data (RGB format)"=w452) -> ("new picture"=w450:picture)  [unwired: 6 in]
      }
    }
    "Elevator View 2" <- w424
    n249 = Index Array(array=w416) -> (element=w415:refnum<vi>)  [unwired: 1 in]
    n250 = property class="DigNum"(reference=w415, "NumText.TextColor"=w414) -> ()  [unwired: 1 in, 2 out]
  }
